vi "Central_Controller_KAFB_v2.vi"() -> ()   [LabVIEW 2019]
uses:
  <vilib>/Modbus/master/Modbus Master.lvclass
  <vilib>/Modbus/master/Create Master Instance (TCP).vi
panel:
  out "randomize 2":u16[](array[numeric])
  out "randomize 1":u16[](array[numeric])
  in  "DER11 Login Button":bool
  in  "DER9 Login Button":bool
  in  "DER7 Login Button":bool
  in  "DER5 Login Button":bool
  in  "DER3 Login Button":bool
  in  "DER2 Login Button":bool
  in  "DER1 Login Button":bool
  in  "DER0 Login Button":bool
  in  "DER4 Login Button":bool
  in  "DER6 Login Button":bool
  in  "DER8 Login Button":bool
  in  "DER10 Login Button":bool
  in  "DER12 Login Button":bool
  in  "DER12 Detail Window Button":bool
  in  "DER11 Detail Window Button":bool
  in  "DER10 Detail Window Button":bool
  in  "DER9 Detail Window Button":bool
  in  "DER8 Detail Window Button":bool
  in  "DER7 Detail Window Button":bool
  in  "DER6 Detail Window Button":bool
  in  "DER2 Detail Window Button":bool
  in  "DER5 Detail Window Button":bool
  in  "DER0 Detail Window Button":bool
  in  "DER1 Detail Window Button":bool
  in  "DER4 Detail Window Button":bool
  in  "DER3 Detail Window Button":bool
  in  "DER1 Control Window Button":bool
  in  "DER11 Control Window Button":bool
  in  "DER9 Control Window Button":bool
  in  "DER7 Control Window Button":bool
  in  "DER2 Control Window Button":bool
  in  "DER5 Control Window Button":bool
  in  "DER0 Control Window Button":bool
  in  "DER3 Control Window Button":bool
  in  "DER4 Control Window Button":bool
  in  "DER6 Control Window Button":bool
  in  "DER8 Control Window Button":bool
  in  "DER10 Control Window Button":bool
  in  "DER12 Control Window Button":bool
  out "ALL Reactive Power":sgl[](array[numeric])
  out "ALL Frequency":sgl[](array[numeric])
  out "ALL Inverter Real Power":sgl[](array[numeric])
  out "ALL Inverter Reactive Power":sgl[](array[numeric])
  out "ALL Generator DC Voltage":sgl[](array[numeric])
  out "ALL Generator DC Current":sgl[](array[numeric])
  out "ALL Solar DC Voltage":sgl[](array[numeric])
  out "ALL Solar DC Current":sgl[](array[numeric])
  in  "DER List":string[](array[string])=["Capstone", "Aquion", "Tesla", "Load Bank", "Motor 1", "Simpliphi 1", "LG Chem", "Outback 1", "Outback 2", "Sunny Island", "ESS", "Fuel Cells", "Sparkplug", "Fronius", "Suny Boy", "Motor 2"]
  out "data":T1
  out "ALL Status":u16[](array[numeric])
  out "SYS Current Time":dbl format="%.3f"
  out "SYS DER Index":i32
  out "ALL Control Method":string[](array[string])
  out "ALL Logged":bool[](array[boolean])
  out "ALL Through Variable":sgl[](array[numeric])
  out "ALL Across Variable":sgl[](array[numeric])
  out "ALL State of Charge":sgl[](array[numeric])
  out "ALL Real Power":sgl[](array[numeric])
  out "ALL Microgrid Voltage":sgl[](array[numeric])
  in  "Tab Control Main":enum32{"Dashboard", "Comms Control"}(tab)
  out "DER1 Level Indicator Figure":dbl(knob) caption="Gauge" scale=-100.0..100.0
  out "DER2 Level Indicator Figure":dbl(knob) caption="Gauge" scale=0.0..100.0
  out "DER3 Level Indicator Figure":dbl(knob) caption="Gauge" scale=0.0..100.0
  out "DER0 State of Charge Figure":sgl(slide) scale=0.0..100.0
  out "DER5 Load Flow":i32(ring)
  out "DER7 Load Flow":i32(ring)
  out "DER9 Load Flow":i32(ring)
  out "DER11 Load Flow":i32(ring)
  out "DER5 Solar Flow":i32(ring)
  out "DER7 Solar Flow":i32(ring)
  out "DER9 Solar Flow":i32(ring)
  out "DER11 Solar Flow":i32(ring)
  out "DER10 status indicator":u32(colorbox)=15263976
  out "DER9 status indicator":u32(colorbox)=15263976
  out "DER8 status indicator":u32(colorbox)=15263976
  out "DER7 status indicator":u32(colorbox)=15263976
  out "DER6 status indicator":u32(colorbox)=15263976
  out "DER5 status indicator":u32(colorbox)=15263976
  out "DER4 status indicator":u32(colorbox)=15263976
  out "DER3 status indicator":u32(colorbox)=15263976
  out "DER2 status indicator":u32(colorbox)=15263976
  out "DER1 status indicator":u32(colorbox)=15263976
  out "DER0 status indicator":u32(colorbox)=15263976
  out "DER11 status indicator 2":u32(colorbox)=15263976
  out "DER12 status indicator":u32(colorbox)=15263976
  out "DER4 Load Flow":i32(ring)
  out "DER6 Load Flow":i32(ring)
  out "DER8 Load Flow":i32(ring)
  out "DER10 Load Flow":i32(ring)
  out "DER4 Solar Flow":i32(ring)
  out "DER6 Solar Flow":i32(ring)
  out "DER8 Solar Flow":i32(ring)
  out "DER10 Solar Flow":i32(ring)
  out "DER12 Load Flow":i32(ring)
  out "DER12 Solar Flow":i32(ring)
  out "DER10 State of Charge Figure":sgl(slide) scale=0.0..100.0
  out "DER12State of Charge Figure":sgl(slide) scale=0.0..100.0
  out "DER4 State of Charge Figure":sgl(slide) scale=0.0..100.0
  out "DER6 State of Charge Figure":sgl(slide) scale=0.0..100.0
  out "DER8 State of Charge Figure":sgl(slide) scale=0.0..100.0
  out "DER12 Solar Power":sgl format="%#.1f"
  out "DER12 Inverter Power":sgl format="%#.1f"
  out "DER11 Solar Power":sgl format="%#.1f"
  out "DER11 Inverter Power":sgl format="%#.1f"
  out "DER10 Solar Power":sgl format="%#.1f"
  out "DER10 Inverter Power":sgl format="%#.1f"
  out "DER9 Solar Power":sgl format="%#.1f"
  out "DER9 Inverter Power":sgl format="%#.1f"
  out "DER8 Solar Power":sgl format="%#.1f"
  out "DER8 Inverter Power":sgl format="%#.1f"
  out "DER7 Solar Power":sgl format="%#.1f"
  out "DER7 Inverter Power":sgl format="%#.1f"
  out "DER6 Solar Power":sgl format="%#.1f"
  out "DER6 Inverter Power":sgl format="%#.1f"
  out "DER5 Solar Power":sgl format="%#.1f"
  out "DER5 Inverter Power":sgl format="%#.1f"
  out "DER4 Solar Power":sgl format="%#.1f"
  out "DER1 Across Variable":sgl format="%#.1f"
  out "DER0 Across Variable":sgl format="%#.1f"
  out "DER12 State of Charge":sgl format="%.1f"
  out "DER12 Real Power":sgl format="%.1f"
  out "DER12 DC Voltage":sgl format="%#.1f"
  out "DER12 AC Line-Line Voltage":sgl=209.57935 format="%.1f"
  out "DER12 State":string
  out "DER11 State of Charge":sgl format="%#.1f"
  out "DER11 Across Variable":sgl format="%#.2f"
  out "DER11 AC Line-Line Votlage":sgl format="%.1f"
  out "DER11 Real Power":sgl format="%.1f"
  out "DER11 State":string
  out "DER10 State of Charge":sgl format="%.1f"
  out "DER10 Real Power":sgl format="%.1f"
  out "DER10 DC Voltage":sgl format="%#.1f"
  out "DER10 AC Line-Line Voltage":sgl=209.57935 format="%.1f"
  out "DER10 State":string
  out "DER9 State of Charge":sgl format="%#.1f"
  out "DER9 Across Variable":sgl format="%#.2f"
  out "DER9 AC Line-Line Votlage":sgl format="%.1f"
  out "DER9 Real Power":sgl format="%.1f"
  out "DER9 State":string
  out "DER8 State of Charge":sgl format="%.1f"
  out "DER8 Real Power":sgl format="%.1f"
  out "DER8 DC Voltage":sgl format="%#.1f"
  out "DER8 AC Line-Line Voltage":sgl=209.57935 format="%.1f"
  out "DER8 State":string
  out "DER7 State of Charge":sgl format="%#.1f"
  out "DER5 State of Charge":sgl format="%#.1f"
  out "DER7 Across Variable":sgl format="%#.2f"
  out "DER7 AC Line-Line Votlage":sgl format="%.1f"
  out "DER7 Real Power":sgl format="%.1f"
  out "DER7 State":string
  out "DER6 State of Charge":sgl format="%.1f"
  out "DER6 Real Power":sgl format="%.1f"
  out "DER6 DC Voltage":sgl format="%#.1f"
  out "DER6 AC Line-Line Voltage":sgl=209.57935 format="%.1f"
  out "DER6 State":string
  out "DER0 State of Charge":sgl format="%.1f"
  out "DER4 State of Charge":sgl format="%.1f"
  out "DER4 Real Power":sgl format="%.1f"
  out "DER4 DC Voltage":sgl format="%#.1f"
  out "DER4 AC Line-Line Voltage":sgl=209.57935 format="%.1f"
  out "DER4 State":string
  out "DER1 Real Power Indicator 1":sgl format="%.1f"
  out "DER1 Reactive Power":sgl format="%#.1f"
  out "DER1 AC Line-Line Voltage":sgl format="%.1f"
  out "DER0 Real Power":sgl format="%#.1f"
  out "DER0 AC Line-Line Voltage":sgl format="%#.1f"
  out "DER2 AC Line-Line Voltage":sgl format="%.1f"
  out "DER2 Real Power":sgl format="%.1f"
  out "DER3 Real Power":sgl format="%#.1f"
  out "DER3 AC Line-Line Votlage":sgl format="%#.1f"
  out "DER5 Across Variable":sgl format="%#.2f"
  out "DER5 AC Line-Line Votlage":sgl format="%.1f"
  out "DER5 Real Power":sgl format="%.1f"
  out "DER0 State":string
  out "DER1 State":string
  out "DER2 State":string
  out "DER3 State":string
  out "DER5 State":string
  out "DER1 Real Power Indicator 2":sgl format="%.1f"
  out "DER1 Frequency":sgl format="%#.1f"
  out "DER4 Inverter Power":sgl format="%#.1f"
  out "DER5 State of Charge Figure":sgl(slide) scale=0.0..100.0
  out "DER7 State of Charge Figure":sgl(slide) scale=0.0..100.0
  out "DER9 State of Charge Figure":sgl(slide) scale=0.0..100.0
  out "DER11 State of Charge Figure":sgl(slide) scale=0.0..100.0
  out "DER12 Flow":u16(ring)
  out "DER11 Flow":u16(ring)
  out "DER10 Flow":u16(ring)
  out "DER9 Flow":u16(ring)
  out "DER8 Flow":u16(ring)
  out "DER7 Flow":u16(ring)
  out "DER6 Flow":u16(ring)
  out "DER5 Flow":u16(ring)
  out "DER4 Flow":u16(ring)
  out "DER3 Flow":u16(ring)
  out "DER2 Flow":u16(ring)
  out "DER0 Flow":u16(ring)
  out "DER1 Flow":u16(ring)
  in  "Container":enum32{"Page 1"}(tab)
  in  "DER Type":string[](array[string])=["Central", "Central", "Central", "Central", "Nanogrid", "Nanogrid", "Nanogrid", "Nanogrid", "Nanogrid", "Nanogrid", "Nanogrid", "Nanogrid", "Nanogrid", "DER13", "DER14", "DER15"]
  out "ALL Error Indicator":bool[](array[boolean])
  out "ALL DER Current Error":errorcluster[](array[cluster])
  out "ALL DER Final Error":errorcluster[](array[cluster])
  in  "IP Address List":string[](array[string])=["10.1.32.65", "10.1.32.32", "10.1.32.95", "10.1.32.97", "10.1.32.45", "10.1.32.67", "10.1.32.70", "10.1.32.100", "10.1.32.69", "10.1.32.38", "10.1.32.43", "10.1.32.75", "10.1.32.74", "10.0.1.192", "10.0.1.207", "10.0.1.196"]
  in  "DER Label Name":string[](array[string])=["DER0", "DER1", "DER2", "DER3", "DER4", "DER5", "DER6", "DER7", "DER8", "DER9", "DER10", "DER11", "DER12", "DER13", "DER14", "DER15"]
  out "SYS Iteration":i32
  in  "stop":bool
  out "SYS Status":string="Reading"
  out "SYS Case":i32
  in  "Read Array":bool[](array[boolean])=[TRUE, TRUE, TRUE, TRUE, TRUE, TRUE, TRUE, TRUE, TRUE, TRUE, TRUE, FALSE, TRUE]
  # "DER0: Heila XX, Sinamics, 10.0.8.XX\nDER1: Heila XX, Socomec, 10.0.8.XX\nDER2: Heila XX, Alencon, 10.0.8.XX\nDER3: Heila XX, Polar Power, 10.0.8.XX\nDER4: Heila XX, Nanogrid 1 \nDER5: Heila XX, Nanogrid 2\nDER6: Heila XX, Nanogrid 3\nDER7: Heila XX, Nanogrid 4 \nDER8: Heila XX, Nanogrid 5\nDER9: Heila XX, Nanogrid 6\nDER10: Heila XX, Nanogrid 7 \nDER11: Heila XX, Nanogrid 8\nDER12: Heila XX, Nanogrid 9"
  # "Nanogrid 5"
  # "Nanogrid 3"
  # "Nanogrid 1"
  # "Nanogrid 9"
  # "Nanogrid 7"
  # "House"
  # "DETL"
  # "Gathering Space"
  # "House"
  # "House"
  # "Battery"
  # "Sinamics + Energport"
  # "Solar"
  # "Load"
  # "Solar"
  # "Load"
  # "Solar"
  # "Load"
  # "Solar"
  # "Load"
  # "Solar"
  # "Load"
  # "kW"
  # "kW"
  # "kW"
  # "kW"
  # "kW"
  # "kW"
  # "kW"
  # "kW"
  # "kW"
  # "kW"
  # "KAFB Microgrid in Real Time"
  # "%"
  # "%"
  # "%"
  # "%"
  # "%"
  # "%"
  # "V"
  # "V"
  # "V"
  # "V"
  # "V"
  # "V"
  # "Inverter"
  # "Utility Grid"
  # "kW"
  # "kW"
  # "kW"
  # "kW"
  # "kW"
  # "kW"
  # "V"
  # "Socomec"
  # "V"
  # "V"
  # "V"
  # "V"
  # "kW"
  # "V"
  # "V"
  # "V ="
  # "V"
  # "f ="
  # "Hz"
  # "P ="
  # "kW"
  # "kW"
  # "kW"
  # "kW"
  # "kW"
  # "kW"
  # "kW"
  # "kVAr"
  # "Q ="
  # "V"
  # "V"
  # "V"
  # "V"
  # "V"
  # "V"
  # "Nanogrid 8"
  # "Nanogrid 6"
  # "Nanogrid 4"
  # "Nanogrid 2"
  # "Solar"
  # "Generators"
  # "Laundry"
  # "House"
  # "House"
  # "EPIC + Polar Power"
  # "House"
  # "PV + Alencon"
  # "Solar"
  # "Load"
  # "Solar"
  # "Load"
  # "Solar"
  # "Load"
  # "Solar"
  # "Load"
  # "kW"
  # "kW"
  # "kW"
  # "kW"
  # "kW"
  # "kW"
  # "kW"
  # "kW"
  # "%"
  # "%"
  # "%"
  # "%"
  # "V"
  # "V"
  # "V"
  # "V"
  # "Program"
  # "Controllable DERs"
  # "DER0: Heila XX, Sinamics, 10.1.32.65\nDER1: Heila XX, Socomec, 10.1.32.32\nDER2: Heila XX, Alencon, 10.1.32.95\nDER3: Heila XX, Polar Power, 10.1.32.97\nDER4: Heila XX, Nanogrid 1, 10.1.32.45 \nDER5: Heila XX, Nanogrid 2, 10.1.32.67\nDER6: Heila XX, Nanogrid 3, 10.1.32.70\nDER7: Heila XX, Nanogrid 4, 10.1.32.100\nDER8: Heila XX, Nanogrid 5, 10.1.32.68\nDER9: Heila XX, Nanogrid 6, 10.1.32.38\nDER10: Heila XX, Nanogrid 7, 10.1.32.43\nDER11: Heila XX, Nanogrid 8\nDER12: Heila XX, Nanogrid 9"
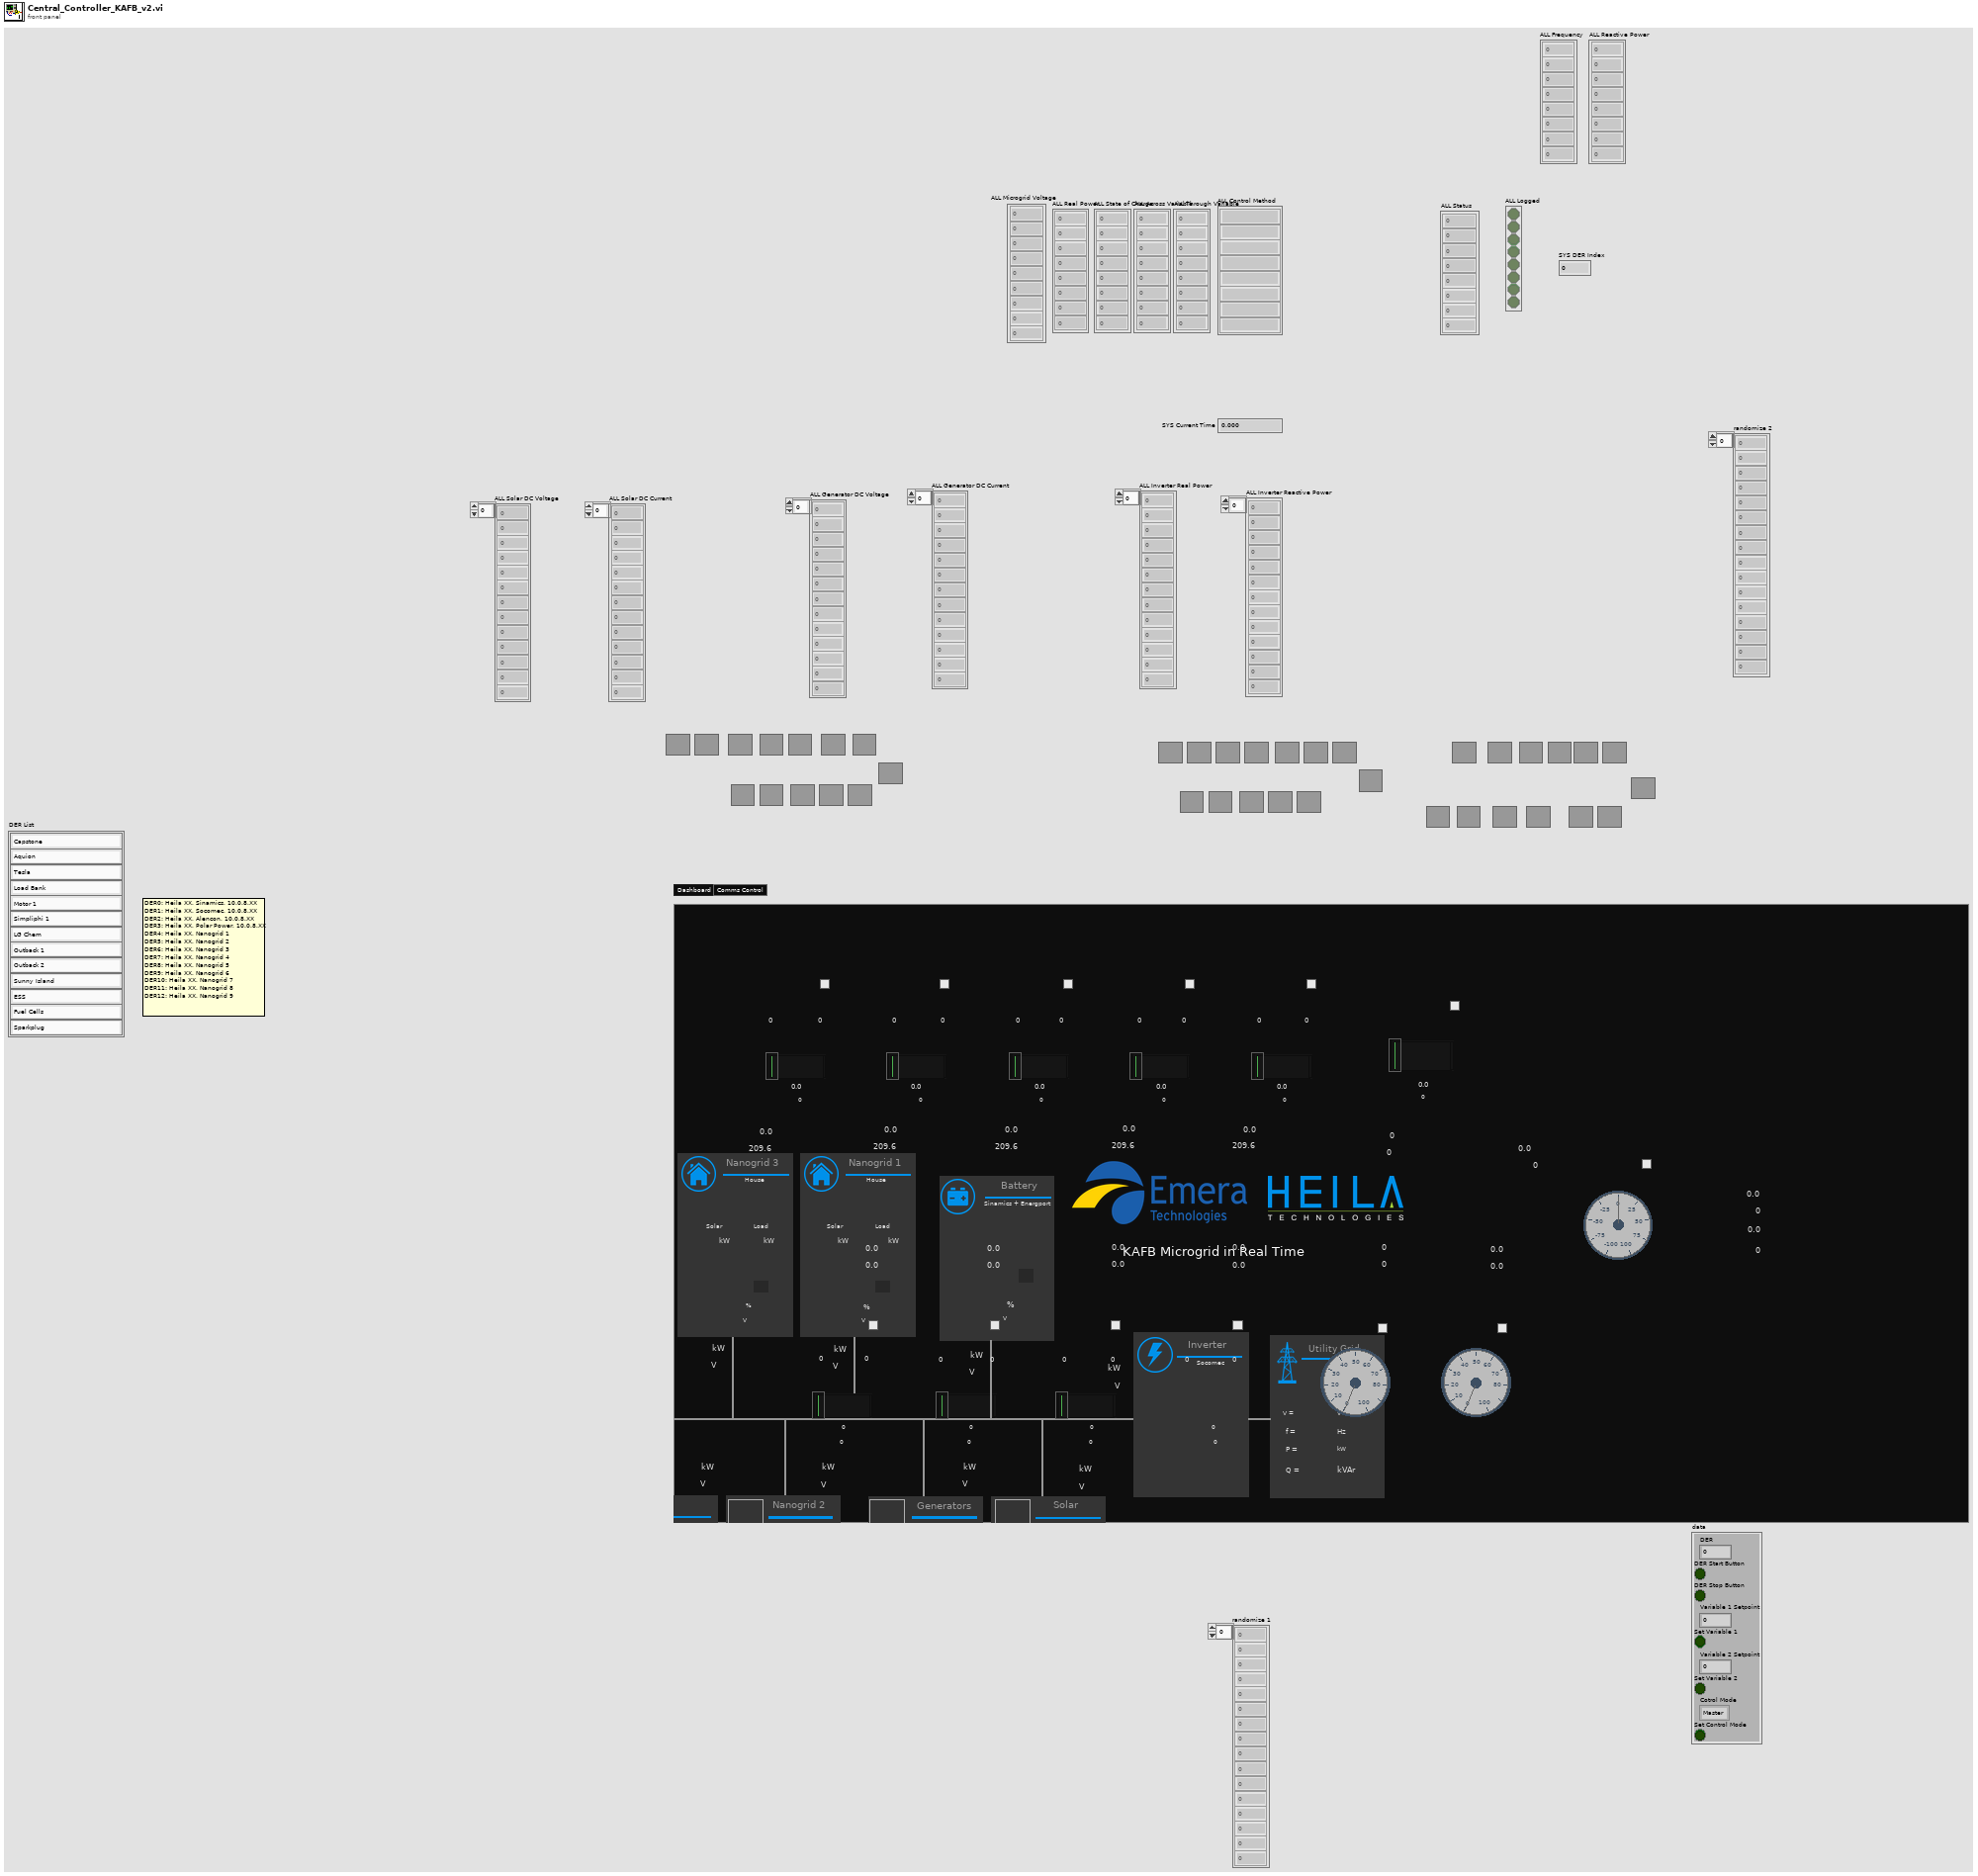
[diagram p1: front panel]
types:
  T1 = cluster{"DER":i32, "DER Start Button":bool, "DER Stop Button":bool, "Variable 1 Setpoint":sgl, "Set Variable 1":bool, "Variable 2 Setpoint":sgl, "Set Variable 2":bool, "Cotrol Mode":enum16{"Master", "Slave"}, "Set Control Mode":bool}
  T2 = cluster{"Modbus master out":refnum<class "Modbus Master.lvclass">, "error out":errorcluster}[]
  T3 = enum32{"Invalid", "Standard", "Closed", "Hidden", "Minimized", "Maximized"}
  T4 = cluster{"Modbus master out":refnum<class "Modbus Master.lvclass">, "error out":errorcluster}
  T5 = enum32{"Bad", "Idle", "Run top level", "Running"}
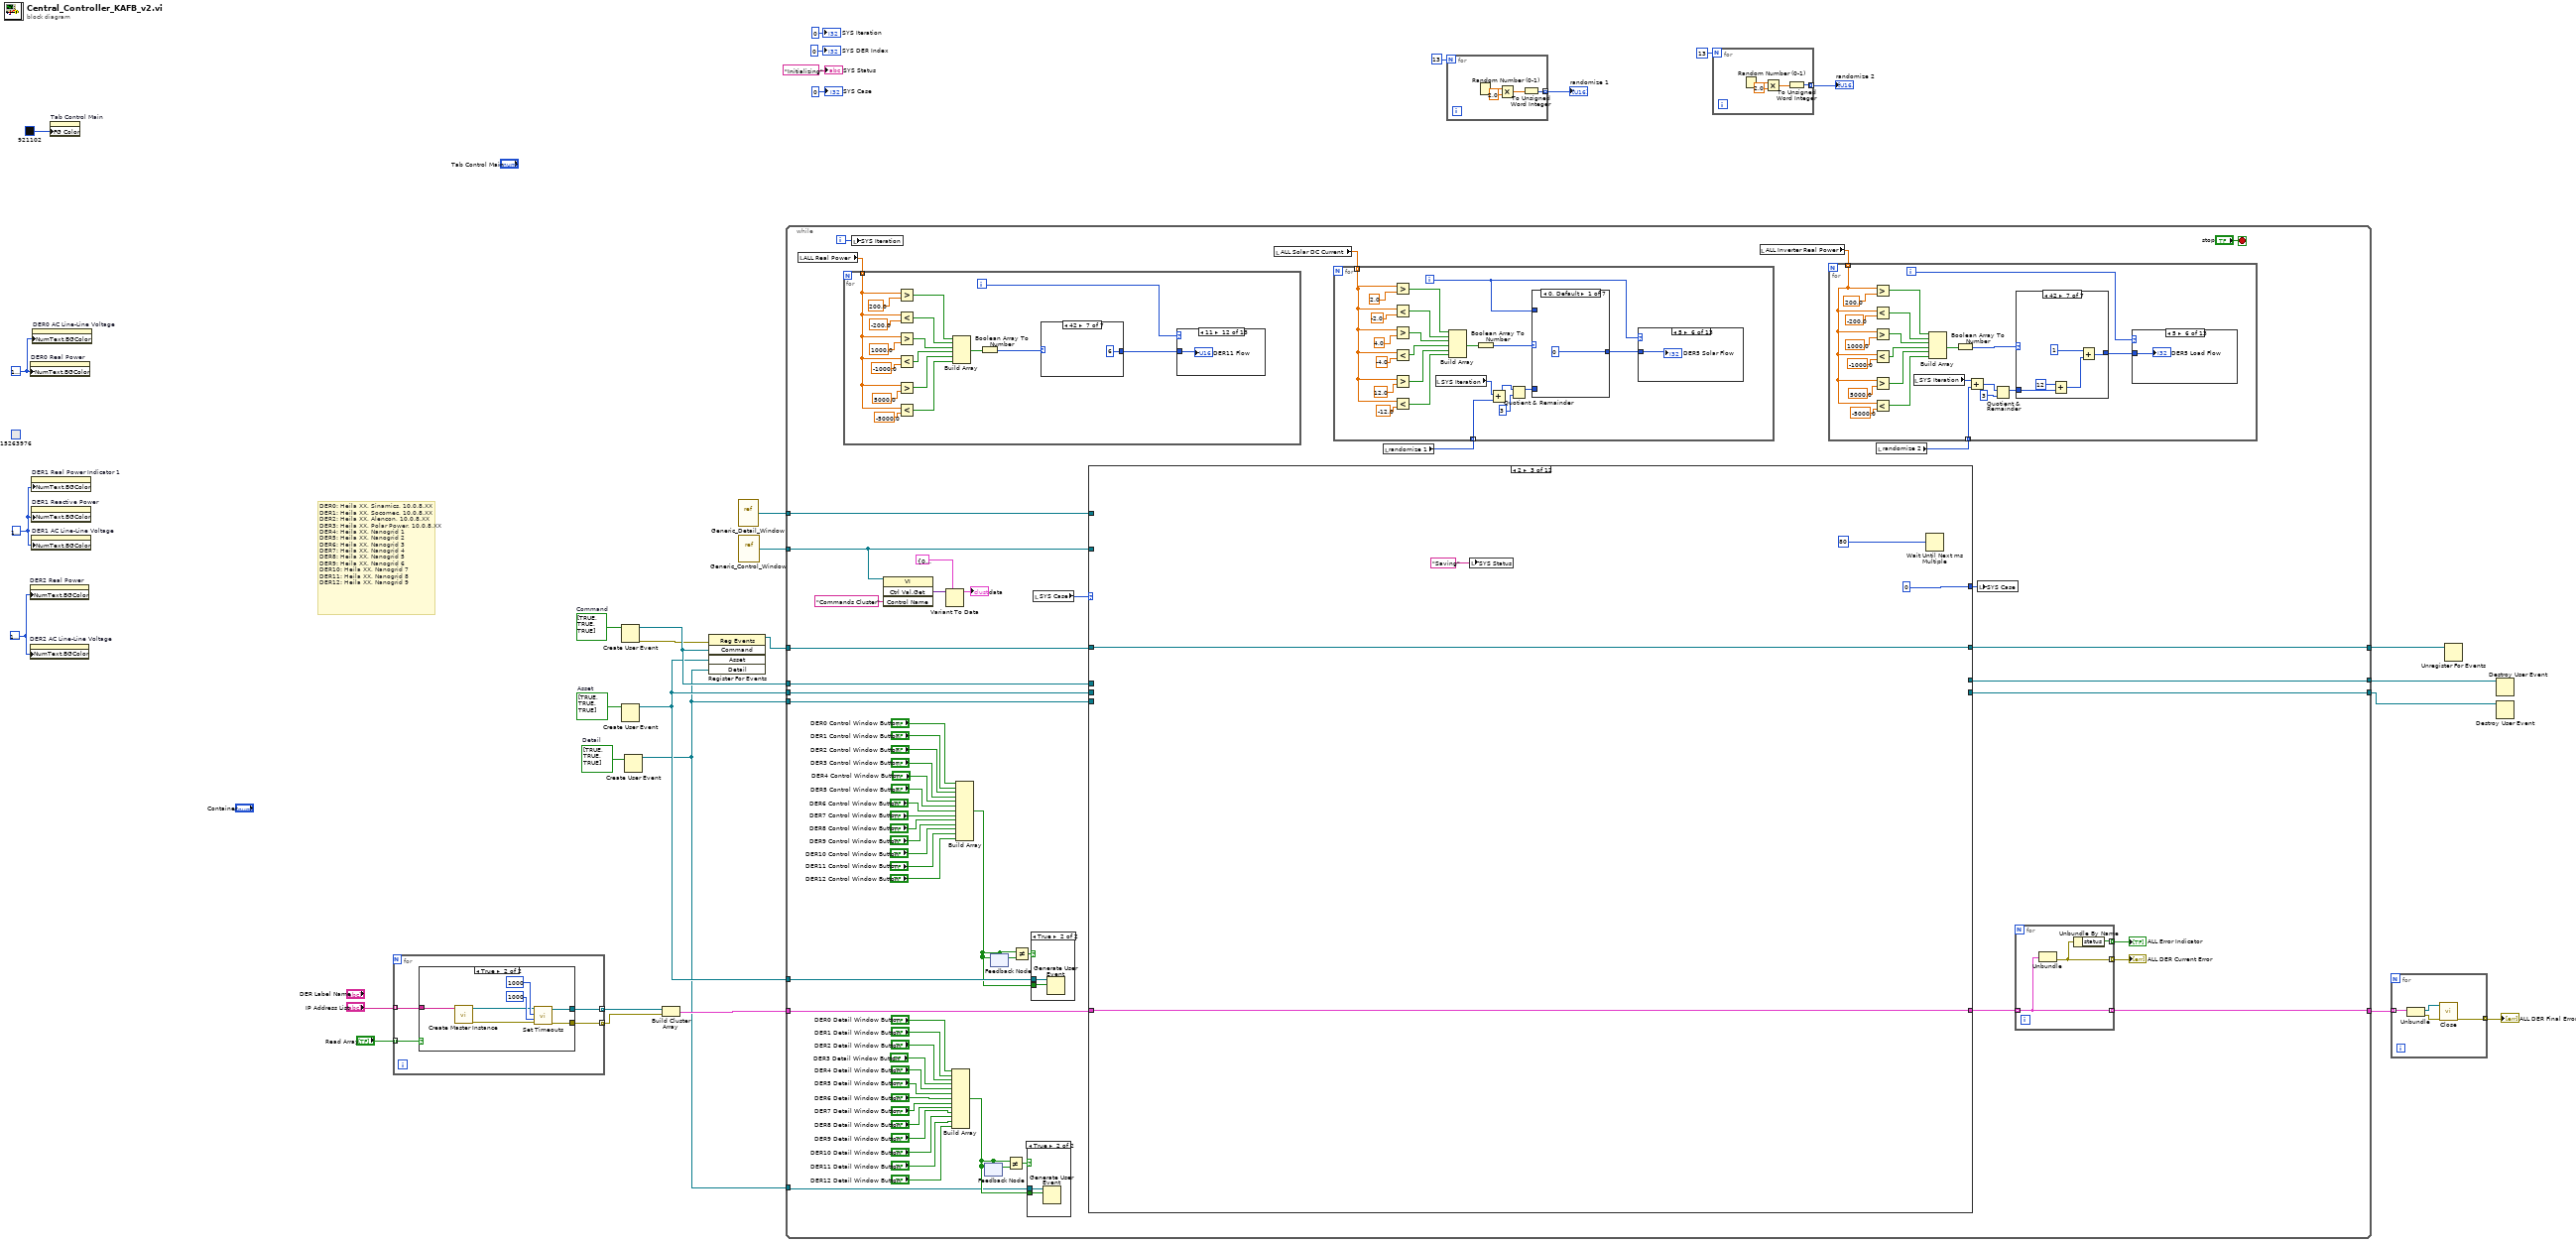
[diagram p0: block diagram]
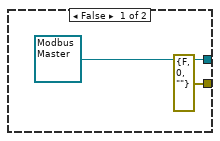
[diagram p2: hidden frame]
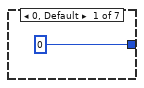
[diagram p3: hidden frame]
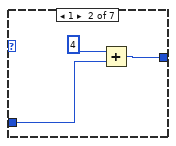
[diagram p4: hidden frame]
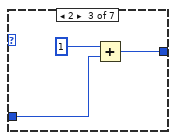
[diagram p5: hidden frame]
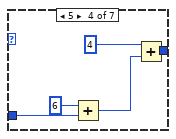
[diagram p6: hidden frame]
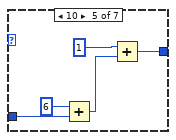
[diagram p7: hidden frame]
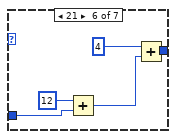
[diagram p8: hidden frame]
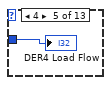
[diagram p13: hidden frame]
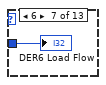
[diagram p14: hidden frame]
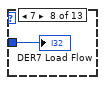
[diagram p15: hidden frame]
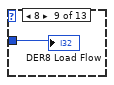
[diagram p16: hidden frame]
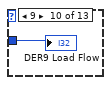
[diagram p17: hidden frame]
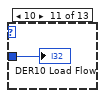
[diagram p18: hidden frame]
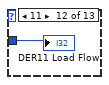
[diagram p19: hidden frame]
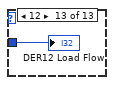
[diagram p20: hidden frame]
diagram:
  w8 = bool[] [TRUE, TRUE, TRUE]  # Detail
  w14 = bool[] [TRUE, TRUE, TRUE]  # Asset
  w17 = bool[] [TRUE, TRUE, TRUE]  # Command
  w28 = u32 16777216
  w29 = u32 16777216
  w30 = u32 16777216
  (unwired) u32 15263976
  # "DER0: Heila XX, Sinamics, 10.0.8.XX\nDER1: Heila XX, Socomec, 10.0.8.XX\nDER2: Heila XX, Alencon, 10.0.8.XX\nDER3: Heila XX, Polar Power, 10.0.8.XX\nDER4: Heila XX, Nanogrid 1 \nDER5: Heila XX, Nanogrid 2\nDER6: Heila XX, Nanogrid 3\nDER7: Heila XX, Nanogrid 4 \nDER8: Heila XX, Nanogrid 5\nDER9: Heila XX, Nanogrid 6\nDER10: Heila XX, Nanogrid 7 \nDER11: Heila XX, Nanogrid 8\nDER12: Heila XX, Nanogrid 9"
  n1 = property on="DER2 Real Power" class="DigNum (strict)"("NumText.BGColor"=w28) -> ()  [unwired: 2 in, 2 out]
  n2 = property on="DER2 AC Line-Line Voltage" class="DigNum (strict)"("NumText.BGColor"=w28) -> ()  [unwired: 2 in, 2 out]
  n3 = property on="DER0 Real Power" class="DigNum (strict)"("NumText.BGColor"=w30) -> ()  [unwired: 2 in, 2 out]
  n4 = property on="DER1 Real Power Indicator 1" class="DigNum (strict)"("NumText.BGColor"=w29) -> ()  [unwired: 2 in, 2 out]
  n5 = property on="DER1 Reactive Power" class="DigNum (strict)"("NumText.BGColor"=w29) -> ()  [unwired: 2 in, 2 out]
  n6 = property on="DER1 AC Line-Line Voltage" class="DigNum (strict)"("NumText.BGColor"=w29) -> ()  [unwired: 2 in, 2 out]
  n7 = property on="DER0 AC Line-Line Voltage" class="DigNum (strict)"("NumText.BGColor"=w30) -> ()  [unwired: 2 in, 2 out]
  n8 = property on="Tab Control Main" class="TabCtl (strict)"("FG Color"=u32 921102) -> ()  [unwired: 2 in, 2 out]
  n9 = for {
    tunnel: "IP Address List" -> [w36] mode=indexing
    tunnel: [w35] -> w27 mode=indexing
    tunnel: [w34] -> w26 mode=indexing
    tunnel: "Read Array" -> [w33] mode=indexing
    n10 = case shown="True" w33 {
      tunnel: w36 -> [_ w45]
      tunnel: [refnum<class "Modbus Master.lvclass"> refnum ("Modbus master out") w42] -> w35
      tunnel: [errorcluster {"status"=FALSE, "code"=0, "source"=""} ("error out") w41] -> w34
      frame False {
      }
      frame True {
        n11 = call-poly <vilib>:"Create Master Instance.vi"("address"=w45) -> ("error out"=w39:errorcluster, "TCP master instance"=w40:refnum<class "Modbus Master.lvclass">)  [unwired: 9 in]
        n12 = call <vilib>:"Set Timeouts.vi"("error in (no error)"=w39, "write operation timeout (ms)"=1000 ("Write Timeout"), "read operation timeout (ms)"=1000 ("Read Timeout"), "Modbus master in"=w40) -> ("error out"=w41:errorcluster, "Modbus master out"=w42:refnum<class "Modbus Master.lvclass">)  [unwired: 6 in]
      }
    }
  }
  n13 = Create User Event(user event datatype=w17) -> (user event=w15:refnum<user-event>, error out=w11:errorcluster)  [unwired: 1 in]
  n14 = Create User Event(user event datatype=w14) -> (user event=w10:refnum<user-event>)  [unwired: 1 in, 1 out]
  n15 = Create User Event(user event datatype=w8) -> (user event=w6:refnum<user-event>)  [unwired: 1 in, 1 out]
  n16 = Build Cluster Array(w27, w26) -> (w25:T2)
  n17 = register-events(error in=w11, w15, w10, w6) -> (reference out=w16:refnum<event-registration>)  [unwired: 1 in, 1 out]
  n18 = vi-ref "Generic_Detail_Window.vi"() -> (w7:refnum<vi>)
  n19 = vi-ref "Generic_Control_Window.vi"() -> (w18:refnum<vi>)
  n20 = while {
    tunnel: w25 -> [w104]
    tunnel: [w100] -> w19
    tunnel: w18 -> [w79]
    tunnel: w15 -> [w97]
    tunnel: w10 -> [w88]
    tunnel: [w85] -> w12
    tunnel: w10 -> [w84]
    tunnel: [w83] -> w9
    tunnel: w16 -> [w98]
    tunnel: [w86] -> w13
    tunnel: w6 -> [w70]
    tunnel: w7 -> [w69]
    tunnel: w6 -> [w68]
    i -> [w51]
    stop <- "stop" stop-if-true
    n21 = local read "ALL Real Power"() -> (w99:sgl[])
    n22 = for {
      tunnel: w99 -> [w232] mode=indexing
      i -> [w237]
      n23 = Greater?(x=w232, y=sgl 200.0) -> (0:w241:bool)
      n24 = Less?(x=w232, y=sgl -200.0) -> (x < y?=w240:bool)
      n25 = Greater?(x=w232, y=sgl 1000.0) -> (0:w231:bool)
      n26 = Less?(x=w232, y=sgl -1000.0) -> (x < y?=w230:bool)
      n27 = Greater?(x=w232, y=sgl 5000.0) -> (0:w229:bool)
      n28 = Less?(x=w232, y=sgl -5000.0) -> (x < y?=w228:bool)
      n29 = Build Array(w241, w240, w231, w230, w229, w228) -> (w239:bool[])
      n30 = Boolean Array To Number(Boolean array=w239) -> (number=w238:u32)
      n31 = case shown="42" w238 {
        tunnel: [0 ("x") 1 ("x") 2 ("x") 3 ("x") 4 ("x") 5 ("x") 6 ("x")] -> w227
        frame 0, Default {
        }
        frame 1 {
        }
        frame 2 {
        }
        frame 5 {
        }
        frame 10 {
        }
        frame 21 {
        }
        frame 42 {
        }
      }
      n32 = case shown="11" w237 {
        tunnel: w227 -> [w251 w252 w253 w254 w255 w256 w257 w258 w259 w260 w261 w262 w263]
        frame 0, Default {
          "DER0 Flow" <- w251
        }
        frame 1 {
          "DER1 Flow" <- w252
        }
        frame 2 {
          "DER2 Flow" <- w253
        }
        frame 3 {
          "DER3 Flow" <- w254
        }
        frame 4 {
          "DER4 Flow" <- w255
        }
        frame 5 {
          "DER5 Flow" <- w256
        }
        frame 6 {
          "DER6 Flow" <- w257
        }
        frame 7 {
          "DER7 Flow" <- w258
        }
        frame 8 {
          "DER8 Flow" <- w259
        }
        frame 9 {
          "DER9 Flow" <- w260
        }
        frame 10 {
          "DER10 Flow" <- w261
        }
        frame 11 {
          "DER11 Flow" <- w262
        }
        frame 12 {
          "DER12 Flow" <- w263
        }
      }
    }
    n33 = local write "SYS Iteration"(w51) -> ()
    n34 = invoke class="VI" method="Ctrl Val.Get"(reference=w79, "Control Name"="Commands Cluster") -> ("Get Control Value Variant"=w96:variant)  [unwired: 2 in, 3 out]
    n35 = Variant To Data(type=T1 {"DER"=0, "DER Start Button"=FALSE, "DER Stop Button"=FALSE, "Variable 1 Setpoint"=0.0, "Set Variable 1"=FALSE, "Variable 2 Setpoint"=0.0, "Set Variable 2"=FALSE, "Cotrol Mode"=enum."Slave", "Set Control Mode"=FALSE} ("Commands Cluster 2"), Variant=w96) -> (data=→"data":T1)  [unwired: 1 in, 1 out]
    n36 = Build Array("DER0 Detail Window Button", "DER1 Detail Window Button", "DER2 Detail Window Button", "DER3 Detail Window Button", "DER4 Detail Window Button", "DER5 Detail Window Button", "DER6 Detail Window Button", "DER7 Detail Window Button", "DER8 Detail Window Button", "DER9 Detail Window Button", "DER10 Detail Window Button", "DER11 Detail Window Button", "DER12 Detail Window Button") -> (w72:bool[])
    n37 = Build Array("DER0 Control Window Button", "DER1 Control Window Button", "DER2 Control Window Button", "DER3 Control Window Button", "DER4 Control Window Button", "DER5 Control Window Button", "DER6 Control Window Button", "DER7 Control Window Button", "DER8 Control Window Button", "DER9 Control Window Button", "DER10 Control Window Button", "DER11 Control Window Button", "DER12 Control Window Button") -> (w87:bool[])
    n38 = feedback #1(w72) -> (w73:bool[])
    n39 = feedback-in #1(w72) -> ()
    n40 = feedback-in #2(w87) -> ()
    n41 = feedback #2(w87) -> (w89:bool[])
    n42 = Not Equal?(x=w72, y=w73) -> (x != y?=w71:bool)
    n43 = Not Equal?(x=w87, y=w89) -> (x != y?=w82:bool)
    n44 = case shown="True" w71 {
      tunnel: w70 -> [_ w224]
      tunnel: w72 -> [_ w223]
      frame False {
      }
      frame True {
        n45 = Generate User Event(user event=w224, event data cluster=w223) -> ()  [unwired: 2 in, 2 out]
      }
    }
    n46 = case shown="True" w82 {
      tunnel: w88 -> [_ w226]
      tunnel: w87 -> [_ w225]
      frame False {
      }
      frame True {
        n47 = Generate User Event(user event=w226, event data cluster=w225) -> ()  [unwired: 2 in, 2 out]
      }
    }
    n48 = local read "SYS Case"() -> (w105:i32)
    n49 = case shown="2" w105 {
      tunnel: [w296 2 0 0 0 0 0 0 0 0 w916 w946] -> w78
      tunnel: [w291 w513 w781 w786 w800 w817 w850 w863 w881 w900 w920 w948] -> w103
      tunnel: w104 -> [w294 w513 w781 w788 w801 w821 w851 w862 w882 w901 w920 w948]
      tunnel: w79 -> [_ _ _ _ _ _ _ _ _ _ w917 _]
      tunnel: w98 -> [w282 w504 w780 _ _ _ _ _ _ _ _ _]
      tunnel: [w281 w504 w780 _ _ _ _ _ _ _ _ _] -> w86
      tunnel: w97 -> [w280 _ _ _ _ _ _ _ _ _ w919 _]
      tunnel: [w280 _ _ _ _ _ _ _ _ _ _ _] -> w85
      tunnel: w84 -> [w279 _ _ _ _ _ _ _ _ _ _ _]
      tunnel: [w279 _ _ _ _ _ _ _ _ _ _ _] -> w83
      tunnel: w69 -> [_ _ _ _ _ _ _ _ _ _ _ w945]
      tunnel: w68 -> [_ _ _ _ _ _ _ _ _ _ _ _]
      frame 0, Default {
        n50 = call "Clock.vi"() -> ("SYS Current Time"=→"SYS Current Time":dbl)  [unwired: 11 in]
        n51 = local read "Read Array"() -> (w277:bool[])
        n52 = for {
          tunnel: w294 -> [w318] mode=indexing
          tunnel: [w317] -> w293 mode=indexing
          tunnel: [w316] -> w292 mode=indexing
          tunnel: [w309] -> w290 mode=indexing
          tunnel: [w315] -> w289 mode=indexing
          tunnel: [w312] -> w288 mode=indexing
          tunnel: [w311] -> w287 mode=indexing
          tunnel: [w314] -> w285 mode=indexing
          tunnel: [w313] -> w286 mode=indexing
          tunnel: [w310] -> w283 mode=indexing
          tunnel: w277 -> [w308] mode=indexing
          tunnel: "DER Type" -> [w307] mode=indexing
          tunnel: [w306] -> w275 mode=indexing
          tunnel: [w305] -> w273 mode=indexing
          tunnel: [w304] -> w274 mode=indexing
          tunnel: [w303] -> w272 mode=indexing
          tunnel: [w302] -> w271 mode=indexing
          tunnel: [w301] -> w270 mode=indexing
          tunnel: [w300] -> w269 mode=indexing
          tunnel: [w299] -> w268 mode=indexing
          tunnel: [w298] -> w267 mode=indexing
          n53 = case shown="True" w308 {
            tunnel: w318 -> [w322 w345]
            tunnel: [w321 w344] -> w317
            tunnel: [w320 w343] -> w316
            tunnel: [w319 w336] -> w315
            tunnel: ["OFF" w342] -> w314
            tunnel: [FALSE w341] -> w313
            tunnel: [w319 w335] -> w312
            tunnel: [w319 w334] -> w311
            tunnel: [u16 1 ("register") w340] -> w310
            tunnel: [w319 w337] -> w309
            tunnel: w307 -> [_ w339]
            tunnel: [w319 w338] -> w306
            tunnel: [w319 w333] -> w305
            tunnel: [w319 w332] -> w304
            tunnel: [w319 w331] -> w303
            tunnel: [w319 w330] -> w302
            tunnel: [w319 w329] -> w301
            tunnel: [w319 w328] -> w300
            tunnel: [w319 w327] -> w299
            tunnel: [w319 w326] -> w298
            frame False {
              w319 = sgl 0.0
              n54 = Unbundle(w322) -> ("Modbus master out"=w321:refnum<class "Modbus Master.lvclass">, "error out"=w320:errorcluster)
            }
            frame True {
              n55 = case shown="\"Central\", Default" w339 {
                tunnel: w345 -> [w393 w431]
                tunnel: [w381 w428] -> w344
                tunnel: [w380 w427] -> w343
                tunnel: [w378 w420] -> w342
                tunnel: [w379 w418] -> w341
                tunnel: [w377 w417] -> w340
                tunnel: [w376 w413] -> w338
                tunnel: [w375 w411] -> w337
                tunnel: [w372 w403] -> w336
                tunnel: [w371 w409] -> w335
                tunnel: [w370 w407] -> w334
                tunnel: [w364 w400] -> w333
                tunnel: [w363 w400] -> w332
                tunnel: [w352 w400] -> w331
                tunnel: [w351 w400] -> w330
                tunnel: [w350 w400] -> w329
                tunnel: [w349 w400] -> w328
                tunnel: [w348 w402] -> w327
                tunnel: [w348 w401] -> w326
                frame "Nanogrid" {
                  w348 = 0.0
                  # "Peripheral 4:\nInverter"
                  # "Peripheral 3:\nGenerator"
                  # "Peripheral 2:\nSolar"
                  # "Peripheral 1:\nBattery"
                  n56 = Unbundle(w393) -> ("Modbus master out"=w395:refnum<class "Modbus Master.lvclass">, "error out"=w394:errorcluster)
                  n57 = call "Read_Electrical_Variables.vi"("error in (no error)"=w394, "Modbus master in"=w395) -> ("error out"=w388:errorcluster, "Variables"=w389:sgl[], "Modbus master out"=w387:refnum<class "Modbus Master.lvclass">)  [unwired: 7 in]
                  n58 = Index Array(array=w389, index #1=7, index #2=10 ("index")) -> (element #1=w376:sgl, element #2=w375:sgl)
                  n59 = call "Read_Electrical_Peripherals.vi"("error in (no error)"=w388, "Peripheral number"=1, "Modbus master in"=w387) -> ("error out"=w365:errorcluster, "Variables"=w374:sgl[], "Modbus master out"=w366:refnum<class "Modbus Master.lvclass">)  [unwired: 6 in]
                  n60 = Index Array(array=w374, index #2=2) -> (element #1=w372:sgl, element #2=w371:sgl, element #3=w370:sgl)  [unwired: 2 in]
                  n61 = call "Read_Electrical_Peripherals.vi"("error in (no error)"=w365, "Peripheral number"=2, "Modbus master in"=w366) -> ("error out"=w357:errorcluster, "Variables"=w368:sgl[], "Modbus master out"=w358:refnum<class "Modbus Master.lvclass">)  [unwired: 6 in]
                  n62 = Index Array(array=w368, index #1=2 ("index")) -> (element #1=w364:sgl, element #2=w363:sgl)  [unwired: 1 in]
                  n63 = call "Read_Electrical_Peripherals.vi"("error in (no error)"=w357, "Peripheral number"=3, "Modbus master in"=w358) -> ("error out"=w355:errorcluster, "Variables"=w361:sgl[], "Modbus master out"=w356:refnum<class "Modbus Master.lvclass">)  [unwired: 6 in]
                  n64 = Index Array(array=w361, index #1=2 ("index")) -> (element #1=w352:sgl, element #2=w351:sgl)  [unwired: 1 in]
                  n65 = call "Read_Electrical_Peripherals.vi"("error in (no error)"=w355, "Peripheral number"=4, "Modbus master in"=w356) -> ("error out"=w346:errorcluster, "Variables"=w353:sgl[], "Modbus master out"=w347:refnum<class "Modbus Master.lvclass">)  [unwired: 6 in]
                  n66 = Index Array(array=w353, index #1=4 ("index")) -> (element #1=w350:sgl, element #2=w349:sgl)  [unwired: 1 in]
                  n67 = call "Read_Status.vi"("error in (no error)"=w346, "Modbus master in"=w347) -> ("error out"=w380:errorcluster, "Variables"=w385:u16[], "Modbus master out"=w381:refnum<class "Modbus Master.lvclass">)  [unwired: 7 in]
                  n68 = Index Array(array=w385, index #3=3) -> (element #1=w377:u16, element #2=w384:u16, element #3=w383:u16)  [unwired: 2 in]
                  n69 = case shown="0, Default" w383 {
                    tunnel: ["Master Mode Simple" "Slave Mode Simple" "Master Mode Droops" "Slave Mode Droops"] -> w378
                    frame 0, Default {
                    }
                    frame 1 {
                    }
                    frame 2 {
                    }
                    frame 3 {
                    }
                  }
                  n70 = Number To Boolean Array(number=w384) -> (Boolean array=w382:bool[])
                  n71 = Index Array(array=w382) -> (element=w379:bool)  [unwired: 1 in]
                }
                frame "Central", Default {
                  w400 = sgl 0.0
                  n72 = Unbundle(w431) -> ("Modbus master out"=w430:refnum<class "Modbus Master.lvclass">, "error out"=w429:errorcluster)
                  n73 = call "Read_Electrical_Variables.vi"("error in (no error)"=w429, "Modbus master in"=w430) -> ("error out"=w415:errorcluster, "Variables"=w425:sgl[], "Modbus master out"=w416:refnum<class "Modbus Master.lvclass">)  [unwired: 7 in]
                  n74 = Index Array(array=w425, index #1=7, index #2=10 ("index"), index #6=17 ("index")) -> (element #1=w413:sgl, element #2=w411:sgl, element #3=w402:sgl, element #5=w401:sgl, element #6=w403:sgl)  [unwired: 3 in, 1 out]
                  n75 = call "Read_Electrical_Peripherals.vi"("error in (no error)"=w415, "Peripheral number"=1, "Modbus master in"=w416) -> ("error out"=w405:errorcluster, "Variables"=w410:sgl[], "Modbus master out"=w406:refnum<class "Modbus Master.lvclass">)  [unwired: 6 in]
                  n76 = Index Array(array=w410, index #1=2) -> (element #1=w409:sgl, element #2=w407:sgl)  [unwired: 1 in]
                  n77 = call "Read_Status.vi"("error in (no error)"=w405, "Modbus master in"=w406) -> ("error out"=w427:errorcluster, "Variables"=w423:u16[], "Modbus master out"=w428:refnum<class "Modbus Master.lvclass">)  [unwired: 7 in]
                  n78 = Index Array(array=w423, index #3=3) -> (element #1=w417:u16, element #2=w422:u16, element #3=w421:u16)  [unwired: 2 in]
                  n79 = case shown="0, Default" w421 {
                    tunnel: ["Master Mode Simple" "Slave Mode Simple" "Master Mode Droops" "Slave Mode Droops"] -> w420
                    frame 0, Default {
                    }
                    frame 1 {
                    }
                    frame 2 {
                    }
                    frame 3 {
                    }
                  }
                  n80 = Number To Boolean Array(number=w422) -> (Boolean array=w419:bool[])
                  n81 = Index Array(array=w419) -> (element=w418:bool)  [unwired: 1 in]
                }
              }
            }
          }
        }
        "ALL Microgrid Voltage" <- w275
        "ALL Real Power" <- w290
        "ALL State of Charge" <- w289
        "ALL Across Variable" <- w288
        "ALL Through Variable" <- w287
        "ALL Logged" <- w286
        "ALL Control Method" <- w285
        "ALL Status" <- w283
        "ALL Solar DC Current" <- w274
        "ALL Solar DC Voltage" <- w273
        "ALL Generator DC Current" <- w271
        "ALL Generator DC Voltage" <- w272
        "ALL Inverter Reactive Power" <- w269
        "ALL Inverter Real Power" <- w270
        "ALL Frequency" <- w268
        "ALL Reactive Power" <- w267
        n82 = local write "SYS Status"("Reading") -> ()
        n83 = event shown="[16] \"DER12 Login Button\": Value Change" {
          selector: w282 -> [w436 _ _ _ w472 _ _ _ _ _ _ _ _ _ _ _ _]
          dyn-events: [w436 _ _ _ w472 _ _ _ _ _ _ _ _ _ _ _ _] -> w281
          timeout: 80 -> [_ _ _ _ _ _ _ _ _ _ _ _ _ _ _ _ _]
          tunnel: [1 w441 w452 w462 13 13 13 13 13 13 13 13 13 13 13 13 13] -> w296
          tunnel: [0 w440 w450 w461 0 1 2 3 4 5 6 7 8 9 10 11 12] -> w284
          event Timeout {
            n84 = event-data() -> ()  [unwired: 1 in, 1 out]
          }
          event User Event {
            n85 = event-data() -> ("Asset"=w445:bool[])  [unwired: 1 in]
            n86 = Search 1D Array(1D array=w445, element=TRUE) -> (index of element=w439:i32)  [unwired: 1 in]
            n87 = Equal?(x=w439, y=-1) -> (x = y?=w442:bool)
            n88 = case shown="False" w442 {
              tunnel: [1000 0] -> w441
              tunnel: [w446 0 ("index of element")] -> w440
              tunnel: w439 -> [w446 _]
              frame False {
              }
              frame True {
              }
            }
          }
          event User Event {
            n89 = event-data() -> ("Command"=w453:bool[])  [unwired: 1 in]
            n90 = Boolean Array To Number(Boolean array=w453) -> (number=w454:u32)
            n91 = case shown="0, Default" w454 {
              tunnel: [0 11 12 14 15 500] -> w452
              frame 0, Default {
              }
              frame 1 {
              }
              frame 2 {
              }
              frame 4 {
              }
              frame 8 {
              }
              frame 16 {
              }
            }
            n92 = local read "data"() -> (w451:T1)
            n93 = Unbundle By Name(w451) -> ("DER"=w450:i32)
          }
          event User Event {
            n94 = event-data() -> ("Detail"=w466:bool[])  [unwired: 1 in]
            n95 = Search 1D Array(1D array=w466, element=TRUE) -> (index of element=w463:i32)  [unwired: 1 in]
            n96 = Equal?(x=w463, y=-1) -> (x = y?=w464:bool)
            n97 = case shown="False" w464 {
              tunnel: [1001 0] -> w462
              tunnel: [w468 0 ("index of element")] -> w461
              tunnel: w463 -> [w468 _]
              frame False {
              }
              frame True {
              }
            }
          }
          event "DER0 Login Button": Value Change {
            n98 = event-data() -> ()  [unwired: 1 in, 1 out]
          }
          event "DER1 Login Button": Value Change {
            n99 = event-data() -> ()  [unwired: 1 in, 1 out]
          }
          event "DER2 Login Button": Value Change {
            n100 = event-data() -> ()  [unwired: 1 in, 1 out]
          }
          event "DER3 Login Button": Value Change {
            n101 = event-data() -> ()  [unwired: 1 in, 1 out]
          }
          event "DER4 Login Button": Value Change {
            n102 = event-data() -> ()  [unwired: 1 in, 6 out]
          }
          event "DER5 Login Button": Value Change {
            n103 = event-data() -> ()  [unwired: 1 in, 1 out]
          }
          event "DER6 Login Button": Value Change {
            n104 = event-data() -> ()  [unwired: 1 in, 6 out]
          }
          event "DER7 Login Button": Value Change {
            n105 = event-data() -> ()  [unwired: 1 in, 6 out]
          }
          event "DER8 Login Button": Value Change {
            n106 = event-data() -> ()  [unwired: 1 in, 6 out]
          }
          event "DER9 Login Button": Value Change {
            n107 = event-data() -> ()  [unwired: 1 in, 6 out]
          }
          event "DER10 Login Button": Value Change {
            n108 = event-data() -> ()  [unwired: 1 in, 6 out]
          }
          event "DER11 Login Button": Value Change {
            n109 = event-data() -> ()  [unwired: 1 in, 6 out]
          }
          event "DER12 Login Button": Value Change {
            n110 = event-data() -> ()  [unwired: 1 in, 6 out]
          }
        }
        n111 = Build Cluster Array(w293, w292) -> (w291:T2)
        n112 = local write "SYS DER Index"(w284) -> ()
      }
      frame 1 {
        # "DER0: Heila XX, Sinamics, 10.0.8.XX\nDER1: Heila XX, Socomec, 10.0.8.XX\nDER2: Heila XX, Alencon, 10.0.8.XX\nDER3: Heila XX, Polar Power, 10.0.8.XX\nDER4: Heila XX, Nanogrid 1 \nDER5: Heila XX, Nanogrid 2\nDER6: Heila XX, Nanogrid 3\nDER7: Heila XX, Nanogrid 4 \nDER8: Heila XX, Nanogrid 5\nDER9: Heila XX, Nanogrid 6\nDER10: Heila XX, Nanogrid 7 \nDER11: Heila XX, Nanogrid 8\nDER12: Heila XX, Nanogrid 9"
        n113 = local read "ALL Solar DC Current"() -> (w500:sgl[])
        n114 = local read "ALL Generator DC Current"() -> (w499:sgl[])
        n115 = local read "ALL Inverter Real Power"() -> (w501:sgl[])
        n116 = local read "ALL Microgrid Voltage"() -> (w512:sgl[])
        n117 = local read "ALL Real Power"() -> (w511:sgl[])
        n118 = local read "ALL Frequency"() -> (w502:sgl[])
        n119 = local read "ALL Reactive Power"() -> (w503:sgl[])
        n120 = local read "ALL State of Charge"() -> (w510:sgl[])
        n121 = local read "ALL Across Variable"() -> (w506:sgl[])
        n122 = local read "ALL Through Variable"() -> (w505:sgl[])
        n123 = local read "ALL Status"() -> (w509:u16[])
        n124 = local read "ALL Logged"() -> (w508:bool[])
        n125 = local read "ALL Control Method"() -> (w507:string[])
        n126 = for {
          tunnel: w512 -> [w530] mode=indexing
          tunnel: w511 -> [w529] mode=indexing
          tunnel: w510 -> [w528] mode=indexing
          tunnel: w509 -> [w523] mode=indexing
          tunnel: w508 -> [w527] mode=indexing
          tunnel: w507 -> [w526] mode=indexing
          tunnel: w506 -> [w525] mode=indexing
          tunnel: w505 -> [w524] mode=indexing
          tunnel: w503 -> [w521] mode=indexing
          tunnel: w502 -> [w520] mode=indexing
          tunnel: w501 -> [w519] mode=indexing
          tunnel: w500 -> [w518] mode=indexing
          tunnel: w499 -> [w517] mode=indexing
          i -> [w531]
          n127 = case shown="7" w523 {
            tunnel: ["Operating" "Off" "Sleeping" "Starting" "Stopping" "Busy" "6: N/A" "Fault" "Standby" "Generic Failure"] -> w522
            frame 0, Default {
            }
            frame 1 {
            }
            frame 2 {
            }
            frame 3 {
            }
            frame 4 {
            }
            frame 5 {
            }
            frame 6 {
            }
            frame 7 {
            }
            frame 8 {
            }
            frame 65535 {
            }
          }
          n128 = case shown="12" w531 {
            tunnel: w530 -> [w546 w563 w578 w591 w610 w630 w650 w670 w690 w710 w730 w753 w772]
            tunnel: w529 -> [w549 w567 w579 w592 w612 w633 w651 w672 w691 w712 w732 w751 w770]
            tunnel: w528 -> [w542 _ _ _ w607 w621 w641 w661 w681 w701 w727 w744 w773]
            tunnel: w527 -> [_ _ _ _ _ _ _ _ _ _ _ _ _]
            tunnel: w526 -> [_ _ _ _ _ _ _ _ _ _ _ _ _]
            tunnel: w525 -> [w545 w562 _ _ w609 w628 w649 w669 w689 w709 w729 w749 w768]
            tunnel: w524 -> [_ _ _ _ _ _ _ _ _ _ _ _ _]
            tunnel: w522 -> [w544 w559 w577 w590 w600 w620 w640 w660 w680 w700 w720 w740 w760]
            tunnel: w521 -> [_ w561 _ _ _ _ _ _ _ _ _ _ _]
            tunnel: w520 -> [_ w560 _ _ _ _ _ _ _ _ _ _ _]
            tunnel: w519 -> [_ _ _ _ w602 w625 w643 w663 w686 w703 w722 w741 w762]
            tunnel: w518 -> [_ _ _ _ w608 w629 w648 w668 w688 w708 w728 w748 w767]
            tunnel: w517 -> [_ _ _ _ _ _ _ _ _ _ _ _ _]
            frame 0, Default {
              n129 = Divide(x=w549, y=sgl 1000.0) -> (x/y=→"DER0 Real Power":sgl)
              n130 = case shown="\"Fault\"" w544 {
                tunnel: [u32 13816530 u32 5025616 u32 9949850 u32 12369084 u32 16777224] -> w543
                frame "Off", Default {
                }
                frame "Operating" {
                }
                frame "Standby" {
                }
                frame "Fault" {
                }
                frame "Busy" {
                }
              }
              "DER0 status indicator" <- w543
              "DER0 AC Line-Line Voltage" <- w546
              "DER0 State" <- w544
              "DER0 State of Charge" <- w542
              "DER0 Across Variable" <- w545
              "DER0 State of Charge Figure" <- w542
            }
            frame 1 {
              n131 = Divide(x=w561, y=sgl 1000.0) -> (x/y=→"DER1 Reactive Power":sgl)
              n132 = Divide(x=w567, y=sgl 1000.0) -> (x/y=w557:sgl)
              "DER1 Real Power Indicator 1" <- w557
              "DER1 Real Power Indicator 2" <- w557
              n133 = case shown="\"Fault\"" w559 {
                tunnel: [u32 13816530 u32 5025616 u32 9949850 u32 12369084 u32 16777224] -> w558
                frame "Off", Default {
                }
                frame "Operating" {
                }
                frame "Standby" {
                }
                frame "Fault" {
                }
                frame "Busy" {
                }
              }
              "DER1 status indicator" <- w558
              n134 = Divide(x=w557, y=sgl 0.66) -> (x/y=→"DER1 Level Indicator Figure":sgl)
              "DER1 AC Line-Line Voltage" <- w563
              "DER1 State" <- w559
              "DER1 Across Variable" <- w562
              "DER1 Frequency" <- w560
            }
            frame 2 {
              n135 = Divide(x=w579, y=sgl 1000.0) -> (x/y=w575:sgl)
              "DER2 Real Power" <- w575
              n136 = case shown="\"Fault\"" w577 {
                tunnel: [u32 13816530 u32 5025616 u32 9949850 u32 12369084 u32 16777224] -> w576
                frame "Off", Default {
                }
                frame "Operating" {
                }
                frame "Standby" {
                }
                frame "Fault" {
                }
                frame "Busy" {
                }
              }
              "DER2 status indicator" <- w576
              n137 = Divide(x=w575, y=sgl 0.4) -> (x/y=→"DER2 Level Indicator Figure":sgl)
              "DER2 AC Line-Line Voltage" <- w578
              "DER2 State" <- w577
            }
            frame 3 {
              n138 = Divide(x=w592, y=1000.0) -> (x/y=w587:dbl)
              "DER3 Real Power" <- w587
              n139 = Divide(x=w587, y=0.24) -> (x/y=→"DER3 Level Indicator Figure":dbl)
              n140 = case shown="\"Fault\"" w590 {
                tunnel: [u32 13816530 u32 5025616 u32 9949850 u32 12369084 u32 16777224] -> w589
                frame "Off", Default {
                }
                frame "Operating" {
                }
                frame "Standby" {
                }
                frame "Fault" {
                }
                frame "Busy" {
                }
              }
              "DER3 status indicator" <- w589
              "DER3 State" <- w590
              "DER3 AC Line-Line Votlage" <- w591
            }
            frame 4 {
              n141 = Divide(x=w612, y=sgl 1000.0) -> (x/y=→"DER4 Real Power":sgl)
              n142 = Multiply(x=w609, y=w608) -> (x*y=w605:sgl)
              n143 = case shown="\"Fault\"" w600 {
                tunnel: [u32 13816530 u32 5025616 u32 9949850 u32 12369084 u32 16777224] -> w599
                frame "Off", Default {
                }
                frame "Operating" {
                }
                frame "Standby" {
                }
                frame "Fault" {
                }
                frame "Busy" {
                }
              }
              "DER4 status indicator" <- w599
              n144 = Divide(x=w605, y=sgl 1000.0) -> (x/y=→"DER4 Solar Power":sgl)
              n145 = Divide(x=w602, y=sgl 1000.0) -> (x/y=→"DER4 Inverter Power":sgl)
              "DER4 DC Voltage" <- w609
              "DER4 AC Line-Line Voltage" <- w610
              "DER4 State" <- w600
              "DER4 State of Charge" <- w607
              "DER4 State of Charge Figure" <- w607
            }
            frame 5 {
              n146 = Divide(x=w633, y=sgl 1000.0) -> (x/y=→"DER5 Real Power":sgl)
              n147 = Multiply(x=w629, y=w628) -> (x*y=w623:sgl)
              n148 = case shown="\"Fault\"" w620 {
                tunnel: [u32 13816530 u32 5025616 u32 9949850 u32 12369084 u32 16777224] -> w619
                frame "Off", Default {
                }
                frame "Operating" {
                }
                frame "Standby" {
                }
                frame "Fault" {
                }
                frame "Busy" {
                }
              }
              "DER5 status indicator" <- w619
              n149 = Divide(x=w623, y=sgl 1000.0) -> (x/y=→"DER5 Solar Power":sgl)
              n150 = Divide(x=w625, y=sgl 1000.0) -> (x/y=→"DER5 Inverter Power":sgl)
              "DER5 Across Variable" <- w628
              "DER5 AC Line-Line Votlage" <- w630
              "DER5 State" <- w620
              "DER5 State of Charge" <- w621
              "DER5 State of Charge Figure" <- w621
            }
            frame 6 {
              n151 = Divide(x=w651, y=sgl 1000.0) -> (x/y=→"DER6 Real Power":sgl)
              n152 = Multiply(x=w649, y=w648) -> (x*y=w646:sgl)
              n153 = case shown="\"Fault\"" w640 {
                tunnel: [u32 13816530 u32 5025616 u32 9949850 u32 12369084 u32 16777224] -> w639
                frame "Off", Default {
                }
                frame "Operating" {
                }
                frame "Standby" {
                }
                frame "Fault" {
                }
                frame "Busy" {
                }
              }
              "DER6 status indicator" <- w639
              n154 = Divide(x=w643, y=sgl 1000.0) -> (x/y=→"DER6 Solar Power":sgl)
              n155 = Divide(x=w646, y=sgl 1000.0) -> (x/y=→"DER6 Inverter Power":sgl)
              "DER6 State" <- w640
              "DER6 AC Line-Line Voltage" <- w650
              "DER6 DC Voltage" <- w649
              "DER6 State of Charge" <- w641
              "DER6 State of Charge Figure" <- w641
            }
            frame 7 {
              n156 = Divide(x=w672, y=sgl 1000.0) -> (x/y=→"DER7 Real Power":sgl)
              n157 = Multiply(x=w669, y=w668) -> (x*y=w666:sgl)
              n158 = case shown="\"Fault\"" w660 {
                tunnel: [u32 13816530 u32 5025616 u32 9949850 u32 12369084 u32 16777224] -> w659
                frame "Off", Default {
                }
                frame "Operating" {
                }
                frame "Standby" {
                }
                frame "Fault" {
                }
                frame "Busy" {
                }
              }
              "DER7 status indicator" <- w659
              n159 = Divide(x=w666, y=sgl 1000.0) -> (x/y=→"DER7 Solar Power":sgl)
              n160 = Divide(x=w663, y=sgl 1000.0) -> (x/y=→"DER7 Inverter Power":sgl)
              "DER7 Across Variable" <- w669
              "DER7 State" <- w660
              "DER7 AC Line-Line Votlage" <- w670
              "DER7 State of Charge" <- w661
              "DER7 State of Charge Figure" <- w661
            }
            frame 8 {
              n161 = Multiply(x=w689, y=w688) -> (x*y=w683:sgl)
              n162 = Divide(x=w691, y=sgl 1000.0) -> (x/y=→"DER8 Real Power":sgl)
              n163 = case shown="\"Fault\"" w680 {
                tunnel: [u32 13816530 u32 5025616 u32 9949850 u32 12369084 u32 16777224] -> w679
                frame "Off", Default {
                }
                frame "Operating" {
                }
                frame "Standby" {
                }
                frame "Fault" {
                }
                frame "Busy" {
                }
              }
              "DER8 status indicator" <- w679
              n164 = Divide(x=w683, y=sgl 1000.0) -> (x/y=→"DER8 Solar Power":sgl)
              n165 = Divide(x=w686, y=sgl 1000.0) -> (x/y=→"DER8 Inverter Power":sgl)
              "DER8 State" <- w680
              "DER8 AC Line-Line Voltage" <- w690
              "DER8 DC Voltage" <- w689
              "DER8 State of Charge" <- w681
              "DER8 State of Charge Figure" <- w681
            }
            frame 9 {
              n166 = Multiply(x=w709, y=w708) -> (x*y=w706:sgl)
              n167 = Divide(x=w712, y=sgl 1000.0) -> (x/y=→"DER9 Real Power":sgl)
              n168 = case shown="\"Fault\"" w700 {
                tunnel: [u32 13816530 u32 5025616 u32 9949850 u32 12369084 u32 16777224] -> w699
                frame "Off", Default {
                }
                frame "Operating" {
                }
                frame "Standby" {
                }
                frame "Fault" {
                }
                frame "Busy" {
                }
              }
              "DER9 status indicator" <- w699
              n169 = Divide(x=w706, y=sgl 1000.0) -> (x/y=→"DER9 Solar Power":sgl)
              n170 = Divide(x=w703, y=sgl 1000.0) -> (x/y=→"DER9 Inverter Power":sgl)
              "DER9 State" <- w700
              "DER9 AC Line-Line Votlage" <- w710
              "DER9 Across Variable" <- w709
              "DER9 State of Charge" <- w701
              "DER9 State of Charge Figure" <- w701
            }
            frame 10 {
              n171 = Multiply(x=w729, y=w728) -> (x*y=w725:sgl)
              n172 = Divide(x=w732, y=sgl 1000.0) -> (x/y=→"DER10 Real Power":sgl)
              n173 = case shown="\"Fault\"" w720 {
                tunnel: [u32 13816530 u32 5025616 u32 9949850 u32 12369084 u32 16777224] -> w719
                frame "Off", Default {
                }
                frame "Operating" {
                }
                frame "Standby" {
                }
                frame "Fault" {
                }
                frame "Busy" {
                }
              }
              "DER10 status indicator" <- w719
              n174 = Divide(x=w722, y=sgl 1000.0) -> (x/y=→"DER10 Inverter Power":sgl)
              n175 = Divide(x=w725, y=sgl 1000.0) -> (x/y=→"DER10 Solar Power":sgl)
              "DER10 State" <- w720
              "DER10 DC Voltage" <- w729
              "DER10 State of Charge" <- w727
              "DER10 AC Line-Line Voltage" <- w730
              "DER10 State of Charge Figure" <- w727
            }
            frame 11 {
              n176 = Divide(x=w751, y=sgl 1000.0) -> (x/y=→"DER11 Real Power":sgl)
              n177 = Multiply(x=w749, y=w748) -> (x*y=w746:sgl)
              n178 = case shown="\"Fault\"" w740 {
                tunnel: [u32 13816530 u32 5025616 u32 9949850 u32 12369084 u32 16777224] -> w739
                frame "Off", Default {
                }
                frame "Operating" {
                }
                frame "Standby" {
                }
                frame "Fault" {
                }
                frame "Busy" {
                }
              }
              "DER11 status indicator 2" <- w739
              n179 = Divide(x=w746, y=sgl 1000.0) -> (x/y=→"DER11 Solar Power":sgl)
              n180 = Divide(x=w741, y=sgl 1000.0) -> (x/y=→"DER11 Inverter Power":sgl)
              "DER11 AC Line-Line Votlage" <- w753
              "DER11 State" <- w740
              "DER11 Across Variable" <- w749
              "DER11 State of Charge" <- w744
              "DER11 State of Charge Figure" <- w744
            }
            frame 12 {
              n181 = Divide(x=w770, y=sgl 1000.0) -> (x/y=→"DER12 Real Power":sgl)
              n182 = Multiply(x=w768, y=w767) -> (x*y=w764:sgl)
              n183 = Divide(x=w762, y=sgl 1000.0) -> (x/y=→"DER12 Inverter Power":sgl)
              n184 = case shown="\"Fault\"" w760 {
                tunnel: [u32 13816530 u32 5025616 u32 9949850 u32 12369084 u32 16777224] -> w759
                frame "Off", Default {
                }
                frame "Operating" {
                }
                frame "Standby" {
                }
                frame "Fault" {
                }
                frame "Busy" {
                }
              }
              "DER12 status indicator" <- w759
              n185 = Divide(x=w764, y=sgl 1000.0) -> (x/y=→"DER12 Solar Power":sgl)
              "DER12 State" <- w760
              "DER12 DC Voltage" <- w768
              "DER12 State of Charge" <- w773
              "DER12State of Charge Figure" <- w773
              "DER12 AC Line-Line Voltage" <- w772
            }
          }
        }
        n186 = local write "SYS Status"("Processing" ("Status")) -> ()
        n187 = Wait Until Next ms Multiple(millisecond multiple=u32 80) -> ()  [unwired: 1 out]
      }
      frame 2 {
        n188 = local write "SYS Status"("Saving" ("Status")) -> ()
        n189 = Wait Until Next ms Multiple(millisecond multiple=u32 80) -> ()  [unwired: 1 out]
      }
      frame 11 {
        n190 = local read "SYS DER Index"() -> (w784:i32)
        n191 = Index Array(array=w788, index=w784) -> (element=w793:T4)
        n192 = Unbundle(w793) -> ("Modbus master out"=w792:refnum<class "Modbus Master.lvclass">, "error out"=w791:errorcluster)
        n193 = local write "SYS Status"("Start" ("Status")) -> ()
        n194 = call-dynamic "Write Single Holding Register.vi"("error in (no error)"=w791, "holding register value"=u16 1, "address"=u16 2032 ("starting address"), "Modbus master in"=w792) -> ("error out"=w789:errorcluster, "Modbus master out"=w790:refnum<class "Modbus Master.lvclass">)  [unwired: 6 in]
        n195 = Bundle("Modbus master out"=w790, "error out"=w789) -> (w787:T4)  [unwired: 1 in]
        n196 = Wait Until Next ms Multiple(millisecond multiple=u32 250) -> ()  [unwired: 1 out]
        n197 = Replace Array Subset(array=w788, new element=w787, index=w784) -> (w786:T2)
      }
      frame 12 {
        n198 = local read "SYS DER Index"() -> (w799:i32)
        n199 = Index Array(array=w801, index=w799) -> (element=w807:T4)
        n200 = Unbundle(w807) -> ("Modbus master out"=w806:refnum<class "Modbus Master.lvclass">, "error out"=w805:errorcluster)
        n201 = local write "SYS Status"("Stop" ("Status")) -> ()
        n202 = call-dynamic "Write Single Holding Register.vi"("error in (no error)"=w805, "holding register value"=u16 0, "address"=u16 2032 ("starting address"), "Modbus master in"=w806) -> ("error out"=w803:errorcluster, "Modbus master out"=w804:refnum<class "Modbus Master.lvclass">)  [unwired: 6 in]
        n203 = Bundle("Modbus master out"=w804, "error out"=w803) -> (w802:T4)  [unwired: 1 in]
        n204 = Replace Array Subset(array=w801, new element=w802, index=w799) -> (w800:T2)
        n205 = Wait Until Next ms Multiple(millisecond multiple=u32 250) -> ()  [unwired: 1 out]
      }
      frame 13 {
        n206 = local read "SYS DER Index"() -> (w812:i32)
        n207 = String To Byte Array(string="HEILA") -> (unsigned byte array=w827:u8[])
        n208 = Index Array(array=w821, index=w812) -> (element=w823:T4)
        n209 = for {
          N: 16 -> [_]
          tunnel: w827 -> [w838]
          tunnel: [w837] -> w815 mode=indexing
          i -> [w833]
          n210 = Multiply(x=w833, y=2) -> (x*y=w834:i32)
          n211 = Increment(x=w834) -> (x+1=w835:i32)
          n212 = Index Array(array=w838, index #1=w834, index #2=w835) -> (element #1=w832:u8, element #2=w830:u8)
          n213 = To Unsigned Byte Integer(number=w832) -> (unsigned 8bit integer=w831:u8)
          n214 = To Unsigned Byte Integer(number=w830) -> (unsigned 8bit integer=w829:u8)
          n215 = Join Numbers(hi=w831, lo=w829) -> ((hi.lo)=w837:u16)
        }
        n216 = Unbundle(w823) -> ("Modbus master out"=w816:refnum<class "Modbus Master.lvclass">, "error out"=w822:errorcluster)
        n217 = call-dynamic "Write Multiple Holding Registers.vi"("error in (no error)"=w822, "holding register values"=w815, "starting address"=u16 2000, "Modbus master in"=w816) -> ("error out"=w819:errorcluster, "Modbus master out"=w820:refnum<class "Modbus Master.lvclass">)  [unwired: 6 in]
        n218 = local write "SYS Status"("Login" ("Status")) -> ()
        n219 = Bundle("Modbus master out"=w820, "error out"=w819) -> (w818:T4)  [unwired: 1 in]
        n220 = Replace Array Subset(array=w821, new element=w818, index=w812) -> (w817:T2)
        n221 = Wait Until Next ms Multiple(millisecond multiple=u32 250) -> ()  [unwired: 1 out]
      }
      frame 14 {
        n222 = local read "SYS DER Index"() -> (w842:i32)
        n223 = Index Array(array=w851, index=w842) -> (element=w852:T4)
        n224 = local read "data"() -> (w839:T1)
        n225 = Unbundle By Name(w839) -> ("Variable 1 Setpoint"=w840:sgl)
        n226 = Type Cast(type=u32 0, x=w840) -> (*(type *) &x=w857:u32)
        n227 = Split Number(x=w857) -> (hi(x)=w855:u16, lo(x)=w854:u16)
        n228 = Unbundle(w852) -> ("Modbus master out"=w849:refnum<class "Modbus Master.lvclass">, "error out"=w848:errorcluster)
        n229 = Build Array(w855, w854) -> (w843:u16[])
        n230 = call-dynamic "Write Multiple Holding Registers.vi"("error in (no error)"=w848, "holding register values"=w843, "starting address"=u16 2036, "Modbus master in"=w849) -> ("error out"=w846:errorcluster, "Modbus master out"=w847:refnum<class "Modbus Master.lvclass">)  [unwired: 6 in]
        n231 = local write "SYS Status"("Set Real Power" ("Status")) -> ()
        n232 = Bundle("Modbus master out"=w847, "error out"=w846) -> (w845:T4)  [unwired: 1 in]
        n233 = Replace Array Subset(array=w851, new element=w845, index=w842) -> (w850:T2)
        n234 = Wait Until Next ms Multiple(millisecond multiple=u32 10) -> ()  [unwired: 1 out]
      }
      frame 15 {
        n235 = local read "SYS DER Index"() -> (w861:i32)
        n236 = local read "data"() -> (w860:T1)
        n237 = Index Array(array=w862, index=w861) -> (element=w871:T4)
        n238 = Unbundle By Name(w860) -> ("Variable 2 Setpoint"=w859:sgl)
        n239 = Type Cast(type=u32 0, x=w859) -> (*(type *) &x=w875:u32)
        n240 = Split Number(x=w875) -> (hi(x)=w873:u16, lo(x)=w872:u16)
        n241 = Unbundle(w871) -> ("Modbus master out"=w870:refnum<class "Modbus Master.lvclass">, "error out"=w869:errorcluster)
        n242 = Build Array(w873, w872) -> (w864:u16[])
        n243 = call-dynamic "Write Multiple Holding Registers.vi"("error in (no error)"=w869, "holding register values"=w864, "starting address"=u16 2038, "Modbus master in"=w870) -> ("error out"=w867:errorcluster, "Modbus master out"=w868:refnum<class "Modbus Master.lvclass">)  [unwired: 6 in]
        n244 = Bundle("Modbus master out"=w868, "error out"=w867) -> (w866:T4)  [unwired: 1 in]
        n245 = Replace Array Subset(array=w862, new element=w866, index=w861) -> (w863:T2)
        n246 = Wait Until Next ms Multiple(millisecond multiple=u32 50) -> ()  [unwired: 1 out]
      }
      frame 16 {
        # "V"
        n247 = local read "SYS DER Index"() -> (w880:i32)
        n248 = local read "data"() -> (w879:T1)
        n249 = Index Array(array=w882, index=w880) -> (element=w890:T4)
        n250 = Unbundle By Name(w879) -> ("Variable 1 Setpoint"=w878:sgl)
        n251 = Type Cast(type=u32 0, x=w878) -> (*(type *) &x=w894:u32)
        n252 = Split Number(x=w894) -> (hi(x)=w892:u16, lo(x)=w891:u16)
        n253 = Unbundle(w890) -> ("Modbus master out"=w889:refnum<class "Modbus Master.lvclass">, "error out"=w888:errorcluster)
        n254 = Build Array(w892, w891) -> (w883:u16[])
        n255 = call-dynamic "Write Multiple Holding Registers.vi"("error in (no error)"=w888, "holding register values"=w883, "starting address"=u16 2040, "Modbus master in"=w889) -> ("error out"=w886:errorcluster, "Modbus master out"=w887:refnum<class "Modbus Master.lvclass">)  [unwired: 6 in]
        n256 = Bundle("Modbus master out"=w887, "error out"=w886) -> (w885:T4)  [unwired: 1 in]
        n257 = Replace Array Subset(array=w882, new element=w885, index=w880) -> (w881:T2)
        n258 = Wait Until Next ms Multiple(millisecond multiple=u32 50) -> ()  [unwired: 1 out]
      }
      frame 17 {
        n259 = local read "SYS DER Index"() -> (w899:i32)
        n260 = local read "data"() -> (w898:T1)
        n261 = Index Array(array=w901, index=w899) -> (element=w909:T4)
        n262 = Unbundle By Name(w898) -> ("Variable 2 Setpoint"=w897:sgl)
        n263 = Type Cast(type=u32 0, x=w897) -> (*(type *) &x=w913:u32)
        n264 = Split Number(x=w913) -> (hi(x)=w911:u16, lo(x)=w910:u16)
        n265 = Unbundle(w909) -> ("Modbus master out"=w908:refnum<class "Modbus Master.lvclass">, "error out"=w907:errorcluster)
        n266 = Build Array(w911, w910) -> (w902:u16[])
        n267 = call-dynamic "Write Multiple Holding Registers.vi"("error in (no error)"=w907, "holding register values"=w902, "starting address"=u16 2042, "Modbus master in"=w908) -> ("error out"=w905:errorcluster, "Modbus master out"=w906:refnum<class "Modbus Master.lvclass">)  [unwired: 6 in]
        n268 = Bundle("Modbus master out"=w906, "error out"=w905) -> (w904:T4)  [unwired: 1 in]
        n269 = Replace Array Subset(array=w901, new element=w904, index=w899) -> (w900:T2)
        n270 = Wait Until Next ms Multiple(millisecond multiple=u32 250) -> ()  [unwired: 1 out]
      }
      frame 1000 {
        n271 = property class="VI"(reference=w917) -> ("Exec.State"=w918:T5)  [unwired: 1 in, 2 out]
        n272 = case shown="\"Idle\"" w918 {
          tunnel: w919 -> [_ w933 _ _]
          tunnel: w917 -> [_ w923 w942 w944]
          tunnel: [0 0 1000 1000] -> w916
          frame "Bad", Default {
          }
          frame "Idle" {
            n273 = invoke class="VI" method="Run VI"(reference=w923, "Wait until done"=FALSE ("Wait Until Done"), "Auto Dispose Ref"=FALSE ("Auto Dispose Reference")) -> (reference out=w929:refnum<vi>)  [unwired: 2 in, 4 out]
            n274 = local read "SYS DER Index"() -> (w936:i32)
            n275 = invoke class="VI" method="FP.Open"(reference=w929, "Activate"=TRUE ("Activate?"), "State"=T3."Standard") -> (reference out=w928:refnum<vi>)  [unwired: 2 in, 4 out]
            n276 = To Variant(anything=w936) -> (Variant=w938:variant)
            n277 = invoke class="VI" method="Ctrl Val.Set"(reference=w928, "Control Name"="DER", "Value"=w938) -> (reference out=w934:refnum<vi>)  [unwired: 2 in, 4 out]
            n278 = To Variant(anything=w933) -> (Variant=w935:variant)
            n279 = invoke class="VI" method="Ctrl Val.Set"(reference=w934, "Control Name"="Event", "Value"=w935) -> (reference out=w925:refnum<vi>)  [unwired: 2 in, 4 out]
            n280 = To Variant(anything="DER List") -> (Variant=w927:variant)
            n281 = invoke class="VI" method="Ctrl Val.Set"(reference=w925, "Control Name"="DER Names", "Value"=w927) -> ()  [unwired: 2 in, 5 out]
          }
          frame "Run top level" {
            n282 = invoke class="VI" method="Abort VI"(reference=w942) -> ()  [unwired: 2 in, 3 out]
          }
          frame "Running" {
            n283 = invoke class="VI" method="Abort VI"(reference=w944) -> ()  [unwired: 2 in, 3 out]
          }
        }
      }
      frame 1001 {
        n284 = property class="VI"(reference=w945) -> ("Exec.State"=w947:T5)  [unwired: 1 in, 2 out]
        n285 = case shown="\"Idle\"" w947 {
          tunnel: w945 -> [_ w956 w966 w968]
          tunnel: [0 0 1000 1000] -> w946
          frame "Bad", Default {
          }
          frame "Idle" {
            n286 = invoke class="VI" method="Run VI"(reference=w956, "Wait until done"=FALSE ("Wait Until Done"), "Auto Dispose Ref"=FALSE ("Auto Dispose Reference")) -> (reference out=w952:refnum<vi>)  [unwired: 2 in, 4 out]
            n287 = local read "SYS DER Index"() -> (w962:i32)
            n288 = invoke class="VI" method="FP.Open"(reference=w952, "Activate"=TRUE ("Activate?"), "State"=T3."Standard") -> (reference out=w953:refnum<vi>)  [unwired: 2 in, 4 out]
            n289 = To Variant(anything=w962) -> (Variant=w964:variant)
            n290 = invoke class="VI" method="Ctrl Val.Set"(reference=w953, "Control Name"="DER", "Value"=w964) -> (reference out=w957:refnum<vi>)  [unwired: 2 in, 4 out]
            n291 = local read "DER List"() -> (w958:string[])
            n292 = To Variant(anything=w958) -> (Variant=w960:variant)
            n293 = invoke class="VI" method="Ctrl Val.Set"(reference=w957, "Control Name"="DER Names", "Value"=w960) -> ()  [unwired: 2 in, 5 out]
          }
          frame "Run top level" {
            n294 = invoke class="VI" method="Abort VI"(reference=w966) -> ()  [unwired: 2 in, 3 out]
          }
          frame "Running" {
            n295 = invoke class="VI" method="Abort VI"(reference=w968) -> ()  [unwired: 2 in, 3 out]
          }
        }
      }
    }
    n296 = local read "ALL Solar DC Current"() -> (w49:sgl[])
    n297 = local read "randomize 1"() -> (w47:u16[])
    n298 = for {
      tunnel: w49 -> [w170] mode=indexing
      tunnel: w47 -> [w167] mode=indexing
      i -> [w169]
      n299 = Greater?(x=w170, y=sgl 2.0) -> (0:w184:bool)
      n300 = Less?(x=w170, y=sgl -2.0) -> (x < y?=w183:bool)
      n301 = Greater?(x=w170, y=sgl 4.0) -> (0:w174:bool)
      n302 = Less?(x=w170, y=sgl -4.0) -> (x < y?=w173:bool)
      n303 = Greater?(x=w170, y=sgl 12.0) -> (0:w172:bool)
      n304 = Less?(x=w170, y=sgl -12.0) -> (x < y?=w171:bool)
      n305 = local read "SYS Iteration"() -> (w166:i32)
      n306 = Build Array(w184, w183, w174, w173, w172, w171) -> (w182:bool[])
      n307 = Boolean Array To Number(Boolean array=w182) -> (number=w181:u32)
      n308 = Add(x=w166, y=w167) -> (x+y=w165:i32)
      n309 = Quotient & Remainder(x=w165, y=3) -> (x-y*floor(x/y)=w179:i32)  [unwired: 1 out]
      n310 = case shown="0, Default" w181 {
        tunnel: [0 ("x") w199 w202 w207 w212 w217 w222] -> w168
        tunnel: w179 -> [_ w198 w201 w206 w210 w215 w220]
        tunnel: w169 -> [_ _ _ _ _ _ _]
        frame 0, Default {
        }
        frame 1 {
          n311 = Add(x=1, y=w198) -> (x+y=w199:i32)
        }
        frame 2 {
          n312 = Add(x=4, y=w201) -> (x+y=w202:i32)
        }
        frame 5 {
          n313 = Add(x=6, y=w206) -> (x+y=w204:i32)
          n314 = Add(x=1, y=w204) -> (x+y=w207:i32)
        }
        frame 10 {
          n315 = Add(x=6, y=w210) -> (x+y=w209:i32)
          n316 = Add(x=4, y=w209) -> (x+y=w212:i32)
        }
        frame 21 {
          n317 = Add(x=12, y=w215) -> (x+y=w214:i32)
          n318 = Add(x=1, y=w214) -> (x+y=w217:i32)
        }
        frame 42 {
          n319 = Add(x=12, y=w220) -> (x+y=w219:i32)
          n320 = Add(x=4, y=w219) -> (x+y=w222:i32)
        }
      }
      n321 = case shown="5" w169 {
        tunnel: w168 -> [_ _ _ _ w187 w188 w189 w190 w191 w192 w193 w194 w195]
        frame 0, Default {
        }
        frame 1 {
        }
        frame 2 {
        }
        frame 3 {
        }
        frame 4 {
          "DER4 Solar Flow" <- w187
        }
        frame 5 {
          "DER5 Solar Flow" <- w188
        }
        frame 6 {
          "DER6 Solar Flow" <- w189
        }
        frame 7 {
          "DER7 Solar Flow" <- w190
        }
        frame 8 {
          "DER8 Solar Flow" <- w191
        }
        frame 9 {
          "DER9 Solar Flow" <- w192
        }
        frame 10 {
          "DER10 Solar Flow" <- w193
        }
        frame 11 {
          "DER11 Solar Flow" <- w194
        }
        frame 12 {
          "DER12 Solar Flow" <- w195
        }
      }
    }
    n322 = local read "ALL Inverter Real Power"() -> (w48:sgl[])
    n323 = local read "randomize 2"() -> (w46:u16[])
    n324 = for {
      tunnel: w48 -> [w114] mode=indexing
      tunnel: w46 -> [w107] mode=indexing
      i -> [w113]
      n325 = Greater?(x=w114, y=sgl 200.0) -> (0:w126:bool)
      n326 = Less?(x=w114, y=sgl -200.0) -> (x < y?=w125:bool)
      n327 = Greater?(x=w114, y=sgl 1000.0) -> (0:w118:bool)
      n328 = Less?(x=w114, y=sgl -1000.0) -> (x < y?=w117:bool)
      n329 = Greater?(x=w114, y=sgl 5000.0) -> (0:w116:bool)
      n330 = Less?(x=w114, y=sgl -5000.0) -> (x < y?=w115:bool)
      n331 = local read "SYS Iteration"() -> (w109:i32)
      n332 = Build Array(w126, w125, w118, w117, w116, w115) -> (w124:bool[])
      n333 = Boolean Array To Number(Boolean array=w124) -> (number=w112:u32)
      n334 = Add(x=w109, y=w107) -> (x+y=w108:i32)
      n335 = Quotient & Remainder(x=w108, y=3) -> (x-y*floor(x/y)=w110:i32)  [unwired: 1 out]
      n336 = case shown="42" w112 {
        tunnel: [0 ("x") w132 w135 w140 w145 w150 w155] -> w111
        tunnel: w110 -> [_ w131 w134 w139 w143 w148 w153]
        frame 0, Default {
        }
        frame 1 {
          n337 = Add(x=4, y=w131) -> (x+y=w132:i32)
        }
        frame 2 {
          n338 = Add(x=1, y=w134) -> (x+y=w135:i32)
        }
        frame 5 {
          n339 = Add(x=6, y=w139) -> (x+y=w137:i32)
          n340 = Add(x=4, y=w137) -> (x+y=w140:i32)
        }
        frame 10 {
          n341 = Add(x=6, y=w143) -> (x+y=w142:i32)
          n342 = Add(x=1, y=w142) -> (x+y=w145:i32)
        }
        frame 21 {
          n343 = Add(x=12, y=w148) -> (x+y=w147:i32)
          n344 = Add(x=4, y=w147) -> (x+y=w150:i32)
        }
        frame 42 {
          n345 = Add(x=12, y=w153) -> (x+y=w152:i32)
          n346 = Add(x=1, y=w152) -> (x+y=w155:i32)
        }
      }
      n347 = case shown="5" w113 {
        tunnel: w111 -> [_ _ _ _ w156 w157 w158 w159 w160 w161 w162 w163 w164]
        frame 0, Default {
        }
        frame 1 {
        }
        frame 2 {
        }
        frame 3 {
        }
        frame 4 {
          "DER4 Load Flow" <- w156
        }
        frame 5 {
          "DER5 Load Flow" <- w157
        }
        frame 6 {
          "DER6 Load Flow" <- w158
        }
        frame 7 {
          "DER7 Load Flow" <- w159
        }
        frame 8 {
          "DER8 Load Flow" <- w160
        }
        frame 9 {
          "DER9 Load Flow" <- w161
        }
        frame 10 {
          "DER10 Load Flow" <- w162
        }
        frame 11 {
          "DER11 Load Flow" <- w163
        }
        frame 12 {
          "DER12 Load Flow" <- w164
        }
      }
    }
    n348 = local write "SYS Case"(w78) -> ()
    n349 = for {
      tunnel: w103 -> [w266] mode=indexing
      tunnel: [w265] -> w102 mode=indexing
      tunnel: [w266] -> w100 mode=indexing
      tunnel: [w264] -> w101 mode=indexing
      n350 = Unbundle(w266) -> ("error out"=w265:errorcluster)  [unwired: 1 out]
      n351 = Unbundle By Name(w265) -> ("status"=w264:bool)
    }
    "ALL DER Current Error" <- w102
    "ALL Error Indicator" <- w101
  }
  n352 = for {
    N: 13 -> [_]
    tunnel: [w969] -> w3 mode=indexing
    n353 = Random Number (0-1)() -> (number: 0 to 1=w972:dbl)
    n354 = Multiply(x=w972, y=2.0) -> (x*y=w970:dbl)
    n355 = To Unsigned Word Integer(number=w970) -> (unsigned 16bit integer=w969:u16)
  }
  "randomize 1" <- w3
  n356 = for {
    N: 13 -> [_]
    tunnel: [w973] -> w1 mode=indexing
    n357 = Random Number (0-1)() -> (number: 0 to 1=w976:dbl)
    n358 = Multiply(x=w976, y=2.0) -> (x*y=w974:dbl)
    n359 = To Unsigned Word Integer(number=w974) -> (unsigned 16bit integer=w973:u16)
  }
  "randomize 2" <- w1
  n360 = for {
    tunnel: w19 -> [w980] mode=indexing
    tunnel: [w977] -> w23 mode=indexing
    n361 = Unbundle(w980) -> ("Modbus master out"=w979:refnum<class "Modbus Master.lvclass">, "error out"=w978:errorcluster)
    n362 = call-dynamic "Close.vi"("error in (no error)"=w978, "Modbus master in"=w979) -> ("error out"=w977:errorcluster)  [unwired: 9 in]
  }
  "ALL DER Final Error" <- w23
  n363 = Unregister For Events(event registration refnum=w13) -> ()  [unwired: 1 in, 1 out]
  n364 = Destroy User Event(user event=w12) -> ()  [unwired: 1 in, 1 out]
  n365 = Destroy User Event(user event=w9) -> ()  [unwired: 1 in, 1 out]
  "SYS Iteration" <- 0
  "SYS DER Index" <- 0 ("DER Index")
  "SYS Status" <- "Initializing" ("Sys Status")
  "SYS Case" <- 0 ("SYS Case")
